vi "pickOffensiveTeam.vi"(0 "OffensiveTeam in":refnum<class "Ally.lvclass">, 1 "Game":refnum<class "Game.lvclass">, 5 "KeeperTeam":refnum<class "Ally.lvclass">, 7 "number_of_robots":i32, 9 "RobotRef":refnum<class "Robot.lvclass">[](array[class]), 11 "error in (no error)":errorcluster) -> (4 "OffensiveTeam out":refnum<class "Ally.lvclass">, 6 "RobotRef":refnum<class "Robot.lvclass">[](array[class]), 15 "error out":errorcluster)   [LabVIEW 2024, in "Ally.lvclass"]
uses:
  Ally.lvclass
  C:/Users/ROBOIME3/Documents/GitHub/SSL_AI/Team_class/Team.lvclass
  Robot_class/Robot.lvclass
  C:/Users/ROBOIME3/Documents/GitHub/SSL_AI/Object_class/Object.lvclass
  Game_class/Game.lvclass
  Utilities_class/Utilities.lvclass
  Team_class/Team.lvclass/Team.ctl
  Team_class/KeeperPlay.ctl
  Team_class/OffensivePlay.ctl
  Game_class/Game.lvclass/Game.ctl
  Parameters_class/Parameters.lvclass/Parameters.ctl
  Events_class/Events.lvclass/Events.ctl
  Object_class/Object.lvclass/Object.ctl
  Ball_class/Ball.lvclass/Ball.ctl
  Robot_class/Robot.lvclass/Robot.ctl
  Controls/AllyTeam.ctl
  Robot_class/roles.ctl
  Zone_class/zones.ctl
  Ally.lvclass/Ally.ctl
  Referee_class/Referee.lvclass/Referee.ctl
  Playbook_class/Playbook.lvclass/Playbook.ctl
  5RobotsSkill_class/5RobotsSkill.lvclass
  EliminateEnum.ctl
  Object_class/Read x.vi
  Object_class/Read y.vi
  Robot_class/Read id.vi
  Team_class/Read RobotRef.vi
  Robot_class/Write role.vi
  Robot_class/Read role.vi
  Robot_class/Write Zone.vi
  Read currentBallZone.vi
  Write currentBallZone.vi
  Game_class/Read Parameters.lvclass.vi
  Game_class/Read Referee.vi
  Referee_class/Read our_goalie_id.vi
  Parameters_class/Read minDistanceToPass.vi
  Playbook_class/Read offensive_plays.vi
  Object_class/Read position(x,y).vi
  Game_class/Read EnemyRef.vi
  Game_class/Read EventsRef.vi
  Game_class/Read BallRef.vi
  Game_class/Read OffensiveTeam.vi
  Game_class/Read NewParameters.vi
  Team_class/Read OffensivePlay.vi
  Ball_class/Read v_x.vi
  Ball_class/Read v_y.vi
  Events_class/Read ball_out_of_vision.vi
  Parameters_class/Read Number of Offesnive.vi
  Team_class/Write RobotRef.vi
  Team_class/Read KeeperPlay.vi
  Ball_class/Ball.lvclass
  Parameters_class/Parameters.lvclass
  Enemy_class/Enemy.lvclass
  Events_class/Events.lvclass
  Playbook_class/Playbook.lvclass
  Play_class/Play.lvclass
  TestPlay_class/TestPlay.lvclass
  EnemyPossessionAtEnemyFieldPlay_class/EnemyPossessionAtEnemyFieldPlay.lvclass
  EnemyPossessionAtOurFieldPlay_class/EnemyPossessionAtOurFieldPlay.lvclass
  NormalGamePlay_class/NormalGamePlay.lvclass
  IndirectEnemyPlay_class/IndirectEnemyPlay.lvclass
  PrepareKickoffAllyPlay_class/PrepareKickoffAllyPlay.lvclass
  PrepareKickoffEnemyPlay_class/PrepareKickoffEnemyPlay.lvclass
  KickPenaltyAllyPlay_class/KickPenaltyAllyPlay.lvclass
  PreparePenaltyAllyPlay_class/PreparePenaltyAllyPlay.lvclass
  DirectEnemyPlay_class/DirectEnemyPlay.lvclass
  PreparePenaltyEnemyPlay_class/PreparePenaltyEnemyPlay.lvclass
  BallOutOfFieldPlay_class/BallOutOfFieldPlay.lvclass
  StopOffensivePlay_class/StopOffensivePlay.lvclass
  PassPlay_class/PassPlay.lvclass
  DirectKickPlay_class/DirectKickPlay.lvclass
  HaltPlay_class/HaltPlay.lvclass
  PreparePassPlay_class/PreparePassPlay.lvclass
  PassToStriker_class/PassToStriker.lvclass
  PassTo2ndStriker_class/PassTo2ndStriker.lvclass
  SimplePass_class/SimplePass.lvclass
  PrepareRollToPassPlay_class/PrepareRollToPassPlay.lvclass
  PrepareDoublePassPlay_class/PrepareDoublePassPlay.lvclass
  TableWith2ndStrikerPlay_class/TableWith2ndStrikerPlay.lvclass
  TableWithStrikerPlay_class/TableWithStrikerPlay.lvclass
  PrepareTriplePassPlay_class/PrepareTriplePassPlay.lvclass
  ABCPassPlay_class/ABCPassPlay.lvclass
  PreparePassInGame1_class/PreparePassInGame1.lvclass
  ACBPassPlay_class/ACBPassPlay.lvclass
  PrepareKeeperPassPlay_class/PrepareKeeperPassPlay.lvclass
  KeeperPassToStrikerPlay_class/KeeperPassToStrikerPlay.lvclass
  5RobotsNormalGamePlay_class/5RobotsNormalGamePlay.lvclass
  5RobotsPassGamePlay_class/5RobotsPassGamePlay.lvclass
  5RobotsKeeperGame_class/5RobotsKeeperGame.lvclass
  5PreparePassGamePlay_class/5PreparePassGamePlay.lvclass
  Referee_class/Referee.lvclass
  Zone_class/Zone.lvclass
  MarkerSkill_class/MarkerSkill.lvclass
  22333355-05bd-4891-b21a-8224ee90334a.vi
  Field_class/Field.lvclass
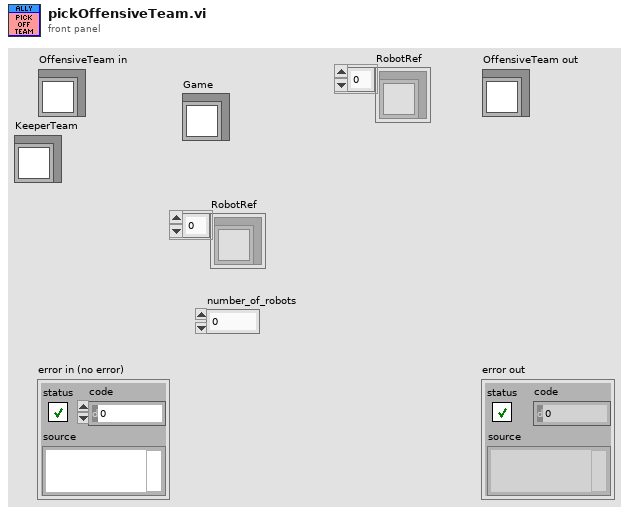
[diagram p1: front panel]
types:
  T1 = typedef "OffensivePlay.ctl" = enum16{"5RobotsPassGamePlay", "5PreparePassGame", "5RobotsKeeperGame", "KeeperPassToStriker", "5RobotsNormalGamePlay", "PrepareKeeperPass", "ACBPass", "ABCPass", "PrepareTriplePass", "TableWithStriker", "TableWith2ndStrikerPlay", "PrepareDoublePass", "PrepareRollToPass", "SimplePass", "PreparePass", "PassToStriker", "BallOutOfField", "PassTo2ndStriker", "StopOffensive", "Prepare Penalty Enemy", "EnemyPossessionAtEnemyField", "EnemyPossesionAtOurField", "TestPlay", "PreparePenaltyAlly", "KickPenaltyAlly", "PrepareKickoffAlly", "PrepareKickoffEnemy", "IndirectEnemy", "DirectEnemy", "PreparePassInGame1", "NormalGame", "DirectKick", "Pass", "Halt", "Timeout", "PassPlay", "PenaltyEnemy"}
  T2 = typedef "KeeperPlay.ctl" = enum16{"SimpleBallPlacementAlly", "BallPlacementAlly", "BallPlacementEnemy", "ZigZag", "Goto", "NormalGame", "KeeperPlay", "Halt", "Timeout", "PenaltyEnemy", "TestPlay"}
  T3 = enum16{"6", "5", "4", "3", "2", "1", "0", "Auto"}
  T4 = typedef "AllyTeam.ctl" = enum16{"Keeper", "Defender", "Attacker"}
  T5 = typedef "roles.ctl" = enum16{"SimpleBallPlacement", "BallPlacementAllyPasser", "BallPlacementAllyReceiver", "BallPlacementEnemy", "5Robots5th", "PassBestReceiver", "5Robots4th", "5Robots3rd", "5Robots2nd", "5Robots1st", "PassBestRobot", "WaitPass", "ABCThirdKicker", "ABCFirstKicker", "ABCSecondKicker", "Tabler", "TableFinalizer", "PrepareRollToPassRoller", "PrepareRollToPassReceiver", "SimplePassRoll", "SimplePassRollReceiver", "PenaltyDefense", "PreparePassReceiver 2", "PreparePassReceiver 1", "PassObserver", "Timeout", "Goto", "ZigZag", "None", "BallOutOfField", "DefenderArea", "Duelist", "AttackerStop", "FollowAttacker", "KeeperRole", "KickPenalty", "AttackerAimGoal", "AttackerBlock", "Marker", "Halt", "Shoot", "PassKicker", "PassReceiver", "TestRole", "PenaltyAttacker"}
  T6 = typedef "EliminateEnum.ctl" = enum16{"0", "1", "2"}
  T7 = typedef "Zone.lvclass/zones.ctl" = enum16{"Field", "LeftSide", "RightSide", "MidField", "LeftForward", "RightForward", "LeftMidField", "RightMidField", "LeftWing", "CenterForward", "RightWing", "Size"}
  T8 = typedef "NewParameters.ctl" = cluster{"PenaltyDistance":dbl, "DistanceAttackerToBackBall":dbl, "Division":enum16{"Div B", "Div A"}, "DistanceToAvoidyEnemyRobot":dbl, "BallPlacementDistance":dbl, "DisatanceBehindBallToStealBall":dbl, "MaxDistanceToPositionKickoff":dbl, "BlockEnemyTarget":bool, "MaxStopVAng":dbl, "DistanceMarkerToEnemy":dbl, "IgnoreDribblerContact":bool, "DistanceToBeginEnemyPosession":dbl, "GoToBallWhenEnemyNotMoving":bool, "EnemyDistanceToReduceVelocity":dbl, "TurnOnEnemyDistanceToReduceVelocity":bool, "EnemyDistanceToShootOutBall":dbl, "DefenseKickBall":bool, "MoreKickToGoal? (0-0.3)":dbl, "ChipKickInEnemyField":bool, "ShootOutRobotId":dbl, "FieldLenghtDenominatorInShootOut":dbl, "AdjustPositionInBallPlacement":bool, "PowerGodPass":dbl, "VelocityAbortEnemyPos":dbl, "MaxDistToBeginPass":dbl, "MinDistToBeginPass":dbl, "VelocityInDirects":dbl, "BadDribblerIDs":i32[], "NewKickToDistanceAroundBall":dbl, "PowerAvoidColisionMarker":dbl, "DistanceToAvoidColisionMarker":dbl, "AvoidBallKick":dbl, "DistanceTryKick":dbl, "SuicideKickDIstance":dbl, "AdjustFirstKickDistance":dbl, "AvoidAimLessKick":dbl, "DistanceToAvoidyEnemyShootRobot ":dbl, "NumberOfMarkers":dbl, "PotField":bool, "PIDLateral":bool, "MinDistanceFirstKickX":dbl, "MinDistanceFirstKickY":dbl, "FractionOfDistToTouchGround\nAfterChipKick":dbl, "FractionOfKickxWhen\nComposedWithKickz":dbl, "Style":T9, "MoveInTurnState":bool, "DistFromEnemyToConsider\nMoveInTurnState":dbl, "CascadePID":bool, "TurnAroundParameters":cluster{"Radius":dbl, "Multiplier":dbl, "ChordAngle":dbl}, "SafeDriveVel":dbl, "DistanceToGoToBackBall":dbl, "minDistanceToNotFinish\nEnemyPossession":dbl, "OneTouchShot":cluster{"angleFactor":dbl, "maxAngle":dbl, "Attack":bool, "Defense":bool}, "OpenAngleToGoal":cluster{"minAngle":dbl, "maxAngle":dbl, "minEvaluation":dbl}, "ShotInterception":cluster{"shotSpeed":dbl, "minEnemySpeed":dbl, "maxEnemySpeed":dbl, "minEvaluation":dbl}, "AllyTeamArray":T4[], "maxDefendersNumber":i32, "Zone":cluster{"GuardPositionArray":dbl[][], "ZoneMidField":dbl[], "CenterForwardWidth":dbl}, "MinEvaluationToShoot":dbl, "PassInterception":cluster{"maxPassSpeed":dbl, "minPassSpeed":dbl, "minEnemySpeed":dbl, "chipPassDistance":dbl, "chipPassEvaluation":dbl, "minEvaluation":dbl, "maxEnemySpeed":dbl}, "PassDistance":cluster{"maxDistance":dbl, "minDistance":dbl}, "receiverSpeed":dbl, "maxBallSpeed":dbl, "slackTime":dbl, "Turning radius":dbl, "Turning v_ang":dbl, "AlignError":cluster{"Distance":dbl, "Orientation":dbl, "V_norm(m/s)":dbl, "V_ang (rad/s)":dbl}, "RobotRadius":dbl, "KickerDistance":dbl, "keeper angle  to cover goalpost":dbl, "a_slide":dbl, "a_roll":dbl, "k_switch":dbl, "Penalty":u16}
  T9 = typedef "Style.ctl" = enum16{"Insanity", "Offensive", "Defensive"}
  T10 = typedef "offensive_plays.ctl" = cluster{"Play":refnum<class "Play.lvclass">, "TestPlay":refnum<class "TestPlay.lvclass">, "EnemyPossessionAtEnemyFieldPlay":refnum<class "EnemyPossessionAtEnemyFieldPlay.lvclass">, "EnemyPossessionAtOurFieldPlay":refnum<class "EnemyPossessionAtOurFieldPlay.lvclass">, "NormalGamePlay":refnum<class "NormalGamePlay.lvclass">, "IndirectEnemyPlay":refnum<class "IndirectEnemyPlay.lvclass">, "PrepareKickoffAllyPlay":refnum<class "PrepareKickoffAllyPlay.lvclass">, "PrepareKickoffEnemyPlay":refnum<class "PrepareKickoffEnemyPlay.lvclass">, "KickPenaltyAllyPlay":refnum<class "KickPenaltyAllyPlay.lvclass">, "PreparePenaltyAllyPlay":refnum<class "PreparePenaltyAllyPlay.lvclass">, "DirectEnemyPlay":refnum<class "DirectEnemyPlay.lvclass">, "PreparePenaltyEnemyPlay":refnum<class "PreparePenaltyEnemyPlay.lvclass">, "BallOutOfFieldPlay":refnum<class "BallOutOfFieldPlay.lvclass">, "StopOffensivePlay":refnum<class "StopOffensivePlay.lvclass">, "PassPlay":refnum<class "PassPlay.lvclass">, "DirectKickPlay":refnum<class "DirectKickPlay.lvclass">, "HaltPlay":refnum<class "HaltPlay.lvclass">, "PreparePassPlay":refnum<class "PreparePassPlay.lvclass">, "PassToStrikerPlay":refnum<class "PassToStriker.lvclass">, "PassTo2ndStrikerPlay":refnum<class "PassTo2ndStriker.lvclass">, "SimplePassPlay":refnum<class "SimplePass.lvclass">, "PrepareRollToPassPlay":refnum<class "PrepareRollToPassPlay.lvclass">, "PrepareDoublePassPlay":refnum<class "PrepareDoublePassPlay.lvclass">, "TableWith2ndStrikerPlay":refnum<class "TableWith2ndStrikerPlay.lvclass">, "TableWithStrikerPlay":refnum<class "TableWithStrikerPlay.lvclass">, "PrepareTriplePassPlay":refnum<class "PrepareTriplePassPlay.lvclass">, "ABCPassPlay":refnum<class "ABCPassPlay.lvclass">, "PreparePassInGame1":refnum<class "PreparePassInGame1.lvclass">, "ACBPassPlay":refnum<class "ACBPassPlay.lvclass">, "PrepareKeeperPassPlay":refnum<class "PrepareKeeperPassPlay.lvclass">, "KeeperPassToStrikerPlay":refnum<class "KeeperPassToStrikerPlay.lvclass">, "SimplePass":refnum<class "SimplePass.lvclass">, "SimplePass 2":refnum<class "SimplePass.lvclass">, "5RobotsNormalGamePlay":refnum<class "5RobotsNormalGamePlay.lvclass">, "5RobotsPassGamePlay":refnum<class "5RobotsPassGamePlay.lvclass">, "5RobotsKeeperGame":refnum<class "5RobotsKeeperGame.lvclass">, "5PreparePassGamePlay":refnum<class "5PreparePassGamePlay.lvclass">}
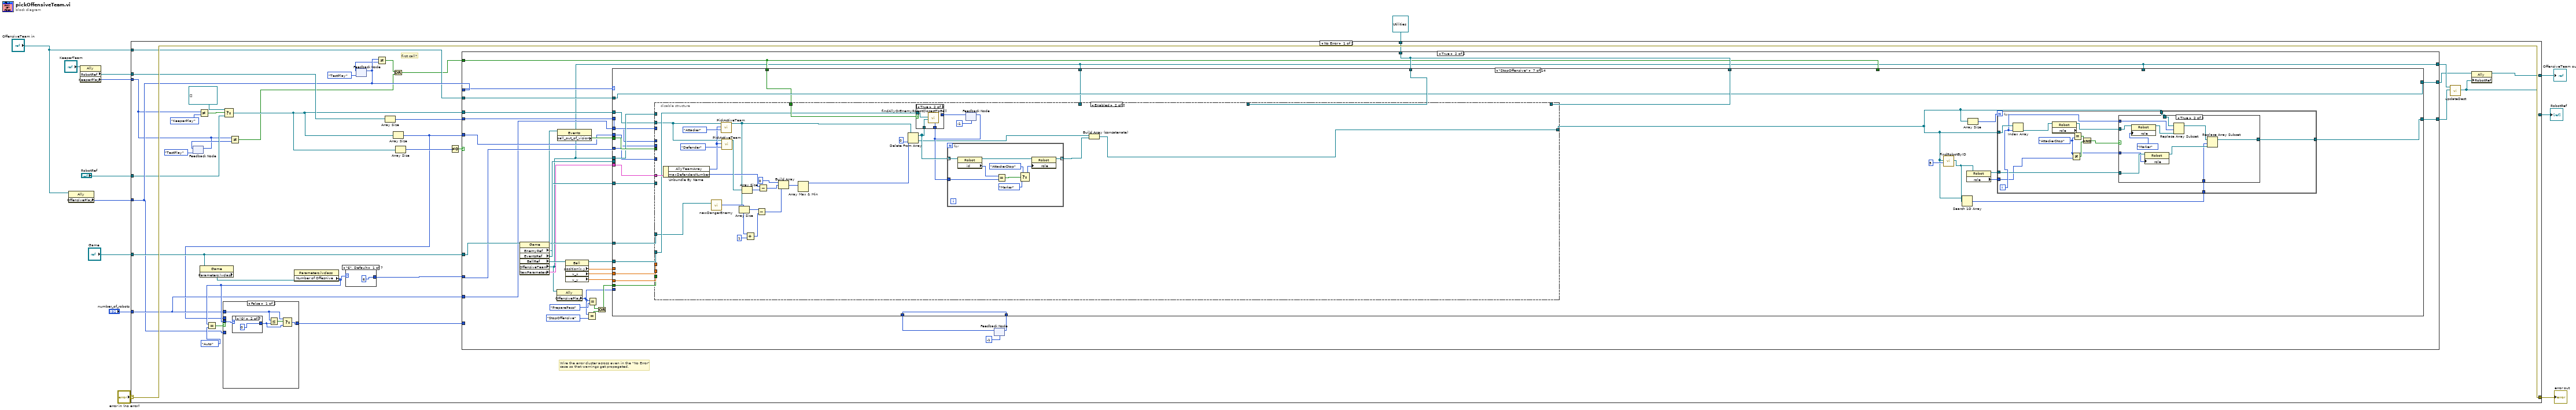
[diagram p0: block diagram]
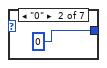
[diagram p2: hidden frame]
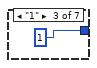
[diagram p3: hidden frame]
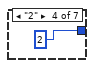
[diagram p4: hidden frame]
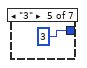
[diagram p5: hidden frame]
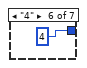
[diagram p6: hidden frame]
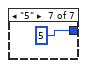
[diagram p7: hidden frame]
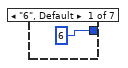
[diagram p8: hidden frame]
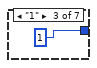
[diagram p9: hidden frame]
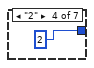
[diagram p10: hidden frame]
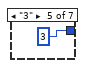
[diagram p11: hidden frame]
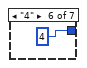
[diagram p12: hidden frame]
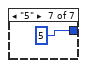
[diagram p13: hidden frame]
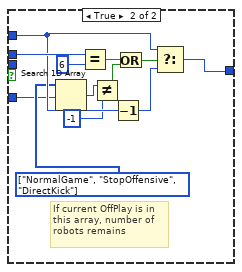
[diagram p14: hidden frame]
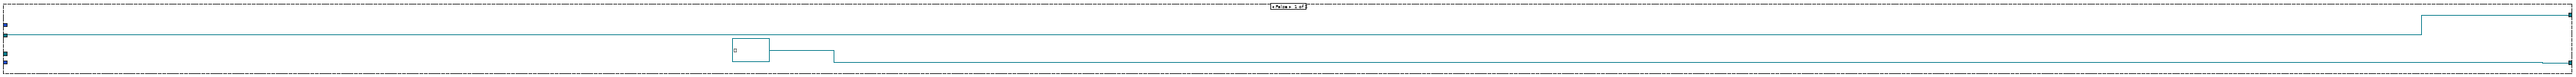
[diagram p15: hidden frame]
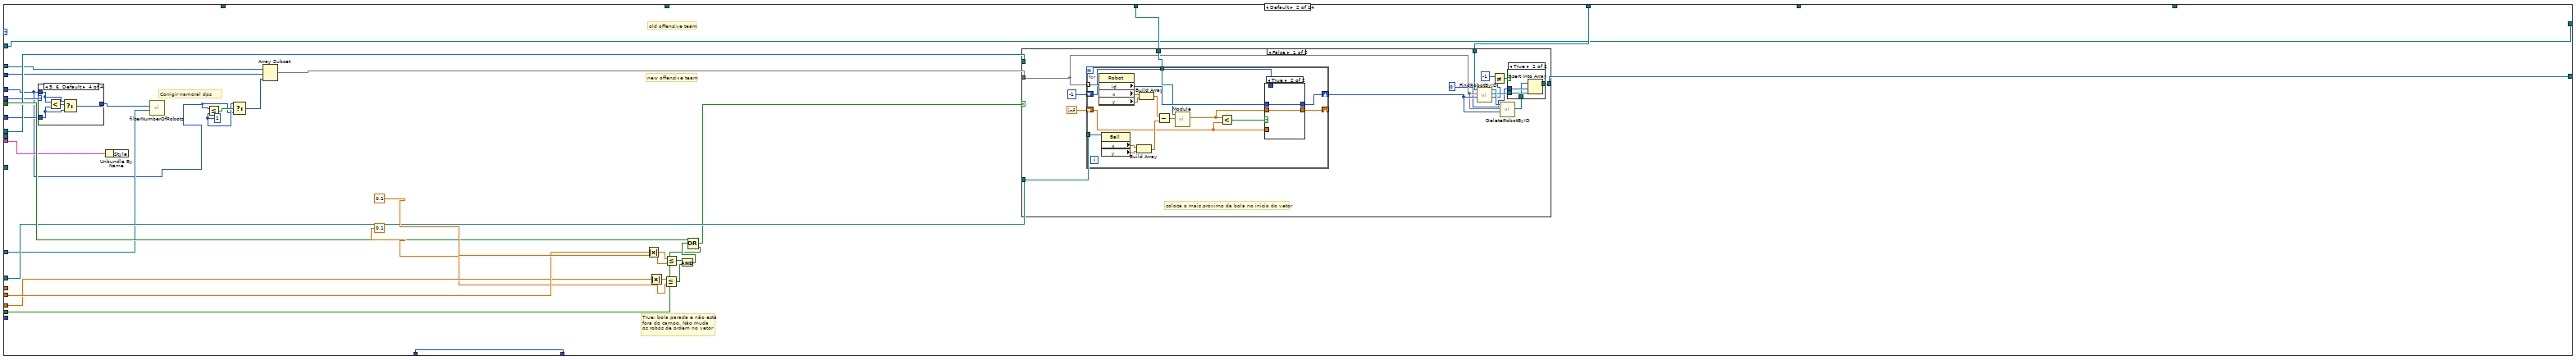
[diagram p17: hidden frame]
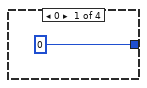
[diagram p18: hidden frame]
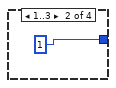
[diagram p19: hidden frame]
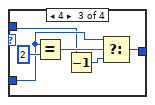
[diagram p20: hidden frame]
diagram:
  n1 = property class="Ally"(reference="OffensiveTeam in") -> ("OffensivePlay"=w2:T1)  [unwired: 1 in, 2 out]
  n2 = property class="Ally"(reference="KeeperTeam") -> ("RobotRef"=w7:refnum<class "Robot.lvclass">[], "KeeperPlay"=w1:T2)  [unwired: 1 in, 2 out]
  n3 = case shown="No Error" "error in (no error)" {
    selector: "error in (no error)" -> [w48 w2386]
    tunnel: [w48 w2386] -> w11
    tunnel: [w47 w2385] -> w13
    tunnel: "OffensiveTeam in" -> [w21 w2385]
    tunnel: "RobotRef" -> [w23 _]
    tunnel: "number_of_robots" -> [w30 _]
    tunnel: w7 -> [w46 _]
    tunnel: [w37 _] -> w6
    tunnel: "Game" -> [w41 _]
    tunnel: refnum<class "Utilities.lvclass"> refnum ("Utilities in") -> [w45 _]
    tunnel: w2 -> [w28 _]
    tunnel: w1 -> [w14 _]
    frame No Error {
      # "first call?"
      # "Wire the error cluster across even in the \"No Error\"\ncase so that warnings get propagated."
      n4 = feedback #1(OffensivePlay."TestPlay" ("OffensivePlay")) -> (w19:u16)
      n5 = feedback-in #1(w14) -> ()
      n6 = Not Equal?(x=w14, y=KeeperPlay."KeeperPlay") -> (x != y?=w24:bool)
      n7 = property class="Game"(reference=w41) -> ("Parameters.lvclass"=w40:refnum<class "Parameters.lvclass">)  [unwired: 1 in, 2 out]
      n8 = Select(t=refnum<class "Robot.lvclass">[] [] ("Array"), s=w24, f=w23) -> (s? t:f=w22:refnum<class "Robot.lvclass">[])
      n9 = Not Equal?(x=w14, y=w19) -> (x != y?=w17:bool)
      n10 = property class="Parameters.lvclass"(reference=w40) -> ("Number of Offesnive"=w32:T3)  [unwired: 1 in, 2 out]
      n11 = Equal?(x=w32, y=T3."Auto") -> (x = y?=w33:bool)
      n12 = case shown="\"6\", Default" w32 {
        tunnel: [6 0 1 2 3 4 5] -> w31
        frame "6", Default {
        }
        frame "0" {
        }
        frame "1" {
        }
        frame "2" {
        }
        frame "3" {
        }
        frame "4" {
        }
        frame "5" {
        }
      }
      n13 = feedback #2(OffensivePlay."TestPlay" ("OffensivePlay")) -> (w27:T1)
      n14 = feedback-in #2(w28) -> ()
      n15 = Not Equal?(x=w28, y=w27) -> (x != y?=w16:bool)
      n16 = Array Size(array=w46) -> (size(s)=w42:i32)
      n17 = Or(x=w16, y=w17) -> (x .or. y?=w15:bool)
      n18 = Array Size(array=w22) -> (size(s)=w29:i32)
      n19 = case shown="False" w33 {
        tunnel: w29 -> [_ w79]
        tunnel: w30 -> [w58 w77]
        tunnel: [w59 w75] -> w38
        tunnel: w32 -> [w60 _]
        tunnel: w28 -> [_ w68]
        frame False {
          n20 = case shown="\"0\"" w60 {
            tunnel: [6 0 1 2 3 4 5] -> w57
            frame "6", Default {
            }
            frame "0" {
            }
            frame "1" {
            }
            frame "2" {
            }
            frame "3" {
            }
            frame "4" {
            }
            frame "5" {
            }
          }
          n21 = Less Or Equal?(x=w58, y=w57) -> (x <= y?=w56:bool)
          n22 = Select(t=w58, s=w56, f=w57) -> (s? t:f=w59:i32)
        }
        frame True {
          w69 = T1[] [enum."NormalGame", enum."StopOffensive", enum."DirectKick"] items=["5RobotsPassGamePlay", "5PreparePassGame", "5RobotsKeeperGame", "KeeperPassToStriker", "5RobotsNormalGamePlay", "PrepareKeeperPass", "ACBPass", "ABCPass", "PrepareTriplePass", "TableWithStriker", "TableWith2ndStrikerPlay", "PrepareDoublePass", "PrepareRollToPass", "SimplePass", "PreparePass", "PassToStriker", "BallOutOfField", "PassTo2ndStriker", "StopOffensive", "Prepare Penalty Enemy", "EnemyPossessionAtEnemyField", "EnemyPossesionAtOurField", "TestPlay", "PreparePenaltyAlly", "KickPenaltyAlly", "PrepareKickoffAlly", "PrepareKickoffEnemy", "IndirectEnemy", "DirectEnemy", "PreparePassInGame1", "NormalGame", "DirectKick", "Pass", "Halt", "Timeout", "PassPlay", "PenaltyEnemy"] ("Array")
          # "If current OffPlay is in\nthis array, number of\nrobots remains"
          n23 = Search 1D Array(1D array=w69, element=w68) -> (index of element=w71:i32)  [unwired: 1 in]
          n24 = Equal?(x=w79, y=6) -> (x = y?=w74:bool)
          n25 = Not Equal?(x=w71, y=-1) -> (x != y?=w72:bool)
          n26 = Decrement(x=w77) -> (x-1=w76:i32)
          n27 = Or(x=w74, y=w72) -> (x .or. y?=w73:bool)
          n28 = Select(t=w77, s=w73, f=w76) -> (s? t:f=w75:i32)
        }
      }
      n29 = Array Size(array=w22) -> (size(s)=w43:i32)
      n30 = Not Equal To 0?(x=w43) -> (x != 0?=w44:bool)
      n31 = case shown="True" w44 {
        tunnel: w38 -> [_ _]
        tunnel: w22 -> [_ w98]
        tunnel: w42 -> [_ w97]
        tunnel: w28 -> [_ w113]
        tunnel: [refnum<class "Robot.lvclass">[] [] w112] -> w36
        tunnel: w41 -> [_ w111]
        tunnel: w45 -> [_ w105]
        tunnel: w15 -> [_ w91]
        tunnel: [_ w82] -> w35
        tunnel: w31 -> [_ w96]
        tunnel: w30 -> [_ w94]
        tunnel: w29 -> [_ w95]
        tunnel: w21 -> [w80 w88]
        tunnel: [w80 w86] -> w20
        frame False {
        }
        frame True {
          n32 = property class="Game"(reference=w111) -> (reference out=w92:refnum<class "Game.lvclass">, "EnemyRef"=w90:refnum<class "Enemy.lvclass">, "EventsRef"=w93:refnum<class "Events.lvclass">, "BallRef"=w110:refnum<class "Ball.lvclass">, "OffensiveTeam"=w82:refnum<class "Ally.lvclass">, "NewParameters"=w89:T8)  [unwired: 1 in, 1 out]
          n33 = property class="Ally"(reference=w82) -> ("OffensivePlay"=w101:T1)  [unwired: 1 in, 2 out]
          n34 = property class="Events"(reference=w93) -> ("ball_out_of_vision"=w107:bool)  [unwired: 1 in, 2 out]
          n35 = property class="Ball"(reference=w110) -> (reference out=w106:refnum<class "Ball.lvclass">, "position(x,y)"=w87:dbl[], "v_x"=w109:dbl, "v_y"=w108:dbl)  [unwired: 1 in, 1 out]
          n36 = Equal?(x=w101, y=OffensivePlay."StopOffensive") -> (x = y?=w99:bool)
          n37 = Equal?(x=w101, y=OffensivePlay."PreparePass") -> (x = y?=w103:bool)
          n38 = Or(x=w103, y=w99) -> (x .or. y?=w102:bool)
          n39 = feedback #3(-1) -> (w84:i32)
          n40 = case shown="\"StopOffensive\"" w113 {
            selector: w113 -> [_ _ _ _ _ _ _ w1611 _ _ w2011 _ _ _]
            tunnel: [w116 w134 w247 w522 w796 w1051 w1295 w1613 w1822 w1912 w2005 w2067 w2143 w2289] -> w112
            tunnel: w109 -> [_ w142 w252 w527 w801 w1056 w1320 _ _ _ _ _ w2162 w2315]
            tunnel: w108 -> [_ w141 w251 w526 w800 w1055 w1319 _ _ _ _ _ w2160 w2313]
            tunnel: w107 -> [_ w138 w250 w525 w799 w1054 w1318 _ _ _ _ _ _ _]
            tunnel: w106 -> [_ w137 w238 w513 w787 w1042 w1307 w1615 w1810 w1913 _ _ w2144 _]
            tunnel: w105 -> [_ w136 w249 w524 w798 w1053 w1317 w1614 _ _ _ _ w2158 w2297]
            tunnel: w105 -> [_ w135 w248 w523 w797 w1052 w1316 _ _ _ _ _ _ _]
            tunnel: w82 -> [_ w133 w246 w521 w795 w1050 w1315 w1607 w1818 w1908 _ _ w2129 _]
            tunnel: w102 -> [_ w132 w245 w520 w794 w1049 w1314 _ _ _ _ _ _ _]
            tunnel: w101 -> [_ _ _ _ _ _ _ _ _ _ _ _ _ _]
            tunnel: w91 -> [_ _ _ _ _ _ _ _ _ _ _ _ w2150 _]
            tunnel: w98 -> [w116 w130 w244 w519 w793 w1048 w1313 w1620 w1823 w1914 w2019 w2080 w2141 w2340]
            tunnel: w97 -> [_ w129 w243 w518 w792 w1047 w1312 w1619 _ _ _ _ _ w2339]
            tunnel: w96 -> [_ w127 w242 w517 w791 w1046 w1311 w1616 _ _ _ _ _ w2336]
            tunnel: w95 -> [_ w126 w241 w516 w790 w1045 w1310 w1617 _ _ _ _ _ w2337]
            tunnel: w94 -> [_ w119 w240 w515 w789 w1044 w1309 w1618 _ _ _ _ _ w2338]
            tunnel: w93 -> [_ _ _ _ _ _ _ _ _ _ _ _ _ _]
            tunnel: w92 -> [_ w121 w237 w512 w786 w1041 w1306 w1612 w1821 w1911 _ _ w2131 w2293]
            tunnel: w91 -> [_ _ w233 w508 _ _ w1302 w1610 _ _ _ _ _ _]
            tunnel: w90 -> [_ _ w239 w514 w788 w1043 w1308 _ _ _ _ _ _ _]
            tunnel: w89 -> [_ w123 w236 w511 w785 w1040 w1305 w1609 w1820 w1910 w2018 w2079 w2140 _]
            tunnel: w88 -> [w115 w118 w235 w510 w784 w1039 w1304 w1608 w1819 w1909 w2010 w2072 w2127 w2285]
            tunnel: w87 -> [_ _ _ _ _ _ _ w1606 w1817 w1907 _ _ _ _]
            tunnel: [w115 w118 w235 w510 w784 w1039 w1304 w1605 w1816 w1906 w2010 w2072 w2126 w2285] -> w86
            tunnel: w84 -> [w114 w117 w234 w509 w783 w1038 w1303 w1604 w1812 w1902 w2009 w2071 w2124 w2284]
            tunnel: [w114 w117 w234 w509 w783 w1038 w1303 w1604 w1813 w1902 w2009 w2071 w2124 w2284] -> w83
            tunnel: w82 -> [_ _ _ _ _ _ _ _ _ _ _ _ _ _]
            tunnel: w82 -> [_ _ _ _ _ _ w1301 _ _ _ _ _ _ _]
            frame "TestPlay" {
              # "Aqui entra a lógica para\nreeordenar o team de acordo \ncom quem deve assumir cada\nrole"
            }
            frame Default {
              w124 = 1 ("y")
              # "Corrigir namoral dps"
              # "old offensive team"
              # "new offensive team"
              # "True: bola parada e não está \nfora do campo. Não muda\nos robôs de ordem no vetor"
              n41 = case shown="5, 6, Default" w126 {
                tunnel: [0 ("number_of_robots") 1 w151 w158] -> w122
                tunnel: w127 -> [_ _ w153 w157]
                tunnel: w119 -> [_ _ w150 w156]
                frame 0 {
                }
                frame 1..3 {
                }
                frame 4 {
                  n42 = Equal?(x=w153, y=2) -> (x = y?=w154:bool)
                  n43 = Decrement(x=w150) -> (x-1=w152:i32)
                  n44 = Select(t=w153, s=w154, f=w152) -> (s? t:f=w151:i32)
                }
                frame 5, 6, Default {
                  n45 = Less?(x=w156, y=w157) -> (x < y?=w159:bool)
                  n46 = Select(t=w156, s=w159, f=w157) -> (s? t:f=w158:i32)
                }
              }
              n47 = Unbundle By Name(w123) -> ()  [unwired: 1 out]
              n48 = call "filterNumberOfRobots.vi"("Game"=w121, "previousNumberOfRobots"=w122) -> ()  [unwired: 7 in, 3 out]
              n49 = Less Or Equal?(x=w119, y=w124) -> (x <= y?=w125:bool)
              n50 = Select(t=w124, s=w125, f=w119) -> (s? t:f=w120:i32)
              n51 = Array Subset(array=w130, index=w129, length=w120) -> (w128:refnum<class "Robot.lvclass">[])
              n52 = Absolute Value(x=w142) -> (abs(x)=w146:dbl)
              n53 = Absolute Value(x=w141) -> (abs(x)=w145:dbl)
              n54 = Less Or Equal?(x=w145, y=0.1) -> (x <= y?=w143:bool)
              n55 = Less Or Equal?(x=w146, y=0.1) -> (x <= y?=w144:bool)
              n56 = Compound Arithmetic op=AND(w144, w143) -> (w139:bool)
              n57 = Compound Arithmetic op=OR(w138, w139, w132) -> (w131:bool)
              n58 = case shown="False" w131 {
                tunnel: w137 -> [w174 _]
                tunnel: w136 -> [w172 w204]
                tunnel: w135 -> [w171 _]
                tunnel: w128 -> [w167 w207]
                tunnel: [w165 w201] -> w134
                tunnel: w133 -> [_ w206]
                frame False {
                  # "coloca o mais próximo da bola no inicio do vetor"
                  n59 = for {
                    tunnel: w167 -> [w196] mode=indexing
                    tunnel: w174 -> [w195]
                    shift-right: [w186] -> w170
                    shift-left: -1 ("id") -> [w182]
                    shift-right: [w184] -> _
                    shift-left: inf -> [w181]
                    tunnel: w172 -> [w180]
                    n60 = property class="Robot"(reference=w196) -> ("id"=w185:i32, "x"=w194:dbl, "y"=w193:dbl)  [unwired: 1 in, 2 out]
                    n61 = property class="Ball"(reference=w195) -> ("x"=w192:dbl, "y"=w191:dbl)  [unwired: 1 in, 2 out]
                    n62 = Build Array(w192, w191) -> (w189:dbl[])
                    n63 = Build Array(w194, w193) -> (w190:dbl[])
                    n64 = Subtract(x=w190, y=w189) -> (x-y=w188:dbl[])
                    n65 = call "Module.vi"("2D vector"=w188, "Utilities in"=w180) -> ("Modulo"=w183:dbl)  [unwired: 7 in, 2 out]
                    n66 = Less?(x=w183, y=w181) -> (x < y?=w187:bool)
                    n67 = case shown="True" w187 {
                      tunnel: [w198 w200] -> w186
                      tunnel: w185 -> [_ w200]
                      tunnel: [w197 w199] -> w184
                      tunnel: w183 -> [_ w199]
                      tunnel: w182 -> [w198 _]
                      tunnel: w181 -> [w197 _]
                      frame False {
                      }
                      frame True {
                      }
                    }
                  }
                  n68 = call "FindRobotByID.vi"("id"=w170, "RobotRef"=w167, "Utilities in"=w171) -> ("index"=w162:i32, "Robot"=w168:refnum<class "Robot.lvclass">, "Utilities out"=w169:refnum<class "Utilities.lvclass">)  [unwired: 5 in, 1 out]
                  n69 = Not Equal?(x=-1, y=w162) -> (x != y?=w160:bool)
                  n70 = call "DeleteRobotByID.vi"("id"=w170, "RobotRef"=w167, "Utilities in"=w169) -> ("RobotRef out"=w164:refnum<class "Robot.lvclass">[])  [unwired: 6 in, 2 out]
                  n71 = case shown="True" w160 {
                    tunnel: w168 -> [_ w179]
                    tunnel: 0 ("index") -> [_ w178]
                    tunnel: [w175 w177] -> w165
                    tunnel: w164 -> [w175 w176]
                    frame False {
                    }
                    frame True {
                      n72 = Insert Into Array(array=w176, index=w178, new element=w179) -> (w177:refnum<class "Robot.lvclass">[])
                    }
                  }
                }
                frame True {
                  n73 = property class="Ally"(reference=w206) -> ("RobotRef"=w205:refnum<class "Robot.lvclass">[])  [unwired: 1 in, 2 out]
                  n74 = for {
                    shift-right: [w209] -> w202
                    shift-left: w207 -> [w212]
                    shift-right: [w210] -> w203
                    shift-left: refnum<class "Robot.lvclass">[] [] -> [w213]
                    tunnel: w205 -> [w214] mode=indexing
                    tunnel: w204 -> [w211]
                    n75 = property class="Robot"(reference=w214) -> ("id"=w219:i32)  [unwired: 1 in, 2 out]
                    n76 = call "FindRobotByID.vi"("id"=w219, "RobotRef"=w212, "Utilities in"=w211) -> ("index"=w216:i32, "Robot"=w220:refnum<class "Robot.lvclass">, "Utilities out"=w218:refnum<class "Utilities.lvclass">)  [unwired: 5 in, 1 out]
                    n77 = Equal?(x=w216, y=-1) -> (x = y?=w217:bool)
                    n78 = case shown="False" w217 {
                      tunnel: w220 -> [w221 _]
                      tunnel: [w227 w229] -> w210
                      tunnel: w213 -> [w226 w229]
                      tunnel: w212 -> [w225 w228]
                      tunnel: w219 -> [w224 _]
                      tunnel: [w223 w228] -> w209
                      tunnel: w218 -> [w222 _]
                      tunnel: w214 -> [_ _]
                      frame False {
                        n79 = Insert Into Array(array=w226, new element=w221) -> (w227:refnum<class "Robot.lvclass">[])  [unwired: 1 in]
                        n80 = call "DeleteRobotByID.vi"("id"=w224, "RobotRef"=w225, "Utilities in"=w222) -> ("RobotRef out"=w223:refnum<class "Robot.lvclass">[])  [unwired: 6 in, 2 out]
                      }
                      frame True {
                      }
                    }
                  }
                  n81 = for {
                    shift-right: [w230] -> w201
                    shift-left: w203 -> [w232]
                    tunnel: w202 -> [w231] mode=indexing
                    n82 = Insert Into Array(array=w232, new element=w231) -> (w230:refnum<class "Robot.lvclass">[])  [unwired: 1 in]
                  }
                }
              }
            }
            frame "EnemyPossesionAtOurField" {
              # "old offensive team"
              n83 = disable-structure shown="Enabled" {
                disable-tunnel: w252 -> [w286 _]
                disable-tunnel: w251 -> [w285 _]
                disable-tunnel: w250 -> [w282 _]
                disable-tunnel: w249 -> [w281 _]
                disable-tunnel: w248 -> [w280 _]
                disable-tunnel: [w279 w485] -> w247
                disable-tunnel: w246 -> [w278 _]
                disable-tunnel: w245 -> [w277 _]
                disable-tunnel: w244 -> [w276 w493]
                disable-tunnel: w243 -> [w275 _]
                disable-tunnel: w242 -> [w273 _]
                disable-tunnel: w241 -> [w272 _]
                disable-tunnel: w240 -> [w271 _]
                disable-tunnel: w239 -> [w270 _]
                disable-tunnel: w238 -> [w268 w468]
                disable-tunnel: w237 -> [w260 w475]
                disable-tunnel: w236 -> [w259 w494]
                disable-tunnel: w233 -> [_ w470]
                frame Disabled {
                  w255 = 1 ("y")
                  # "Deve trocar quem vai pra bola\nquando trocar robô inimigo mais\nperto da bola"
                  # "new offensive team"
                  # "True: bola parada e não está \nfora do campo. Não muda\nos robôs de ordem no vetor"
                  n84 = case shown="0" w272 {
                    tunnel: [0 ("number_of_robots") 1 w295 w302] -> w261
                    tunnel: w273 -> [_ _ w297 w301]
                    tunnel: w271 -> [_ _ w294 w300]
                    frame 0 {
                    }
                    frame 1..3 {
                    }
                    frame 4 {
                      n85 = Equal?(x=w297, y=2) -> (x = y?=w298:bool)
                      n86 = Decrement(x=w294) -> (x-1=w296:i32)
                      n87 = Select(t=w297, s=w298, f=w296) -> (s? t:f=w295:i32)
                    }
                    frame 5, 6, Default {
                      n88 = Less?(x=w300, y=w301) -> (x < y?=w303:bool)
                      n89 = Select(t=w300, s=w303, f=w301) -> (s? t:f=w302:i32)
                    }
                  }
                  n90 = Unbundle By Name(w259) -> ("Style"=w257:T9)
                  n91 = property class="Enemy"(reference=w270) -> ("RobotRef"=w269:refnum<class "Robot.lvclass">[])  [unwired: 1 in, 2 out]
                  n92 = call "filterNumberOfRobots.vi"("Game"=w260, "previousNumberOfRobots"=w261) -> ("finalNumberOfRobots"=w258:i32)  [unwired: 7 in, 2 out]
                  n93 = call "findAllyOrEnemyRobotClosestToBall.vi"("Ally/Enemy Robots"=w269, "Ball"=w268) -> ("Robot"=w267:refnum<class "Robot.lvclass">)  [unwired: 5 in, 4 out]
                  n94 = Subtract(x=w258, y=w257) -> (x-y=w254:i32)
                  n95 = Less Or Equal?(x=w254, y=w255) -> (x <= y?=w256:bool)
                  n96 = Select(t=w255, s=w256, f=w254) -> (s? t:f=w253:i32)
                  n97 = Array Subset(array=w276, index=w275, length=w253) -> (w274:refnum<class "Robot.lvclass">[])
                  n98 = property class="Robot"(reference=w267) -> (reference out=w262:refnum<class "Robot.lvclass">, "id"=w264:i32)  [unwired: 1 in, 1 out]
                  n99 = feedback #4(-1) -> (w266:i32)
                  n100 = Not Equal?(x=w264, y=w266) -> (x != y?=w263:bool)
                  n101 = feedback-in #4(w264) -> ()
                  n102 = Absolute Value(x=w286) -> (abs(x)=w290:dbl)
                  n103 = Absolute Value(x=w285) -> (abs(x)=w289:dbl)
                  n104 = Less Or Equal?(x=w289, y=0.1) -> (x <= y?=w287:bool)
                  n105 = Less Or Equal?(x=w290, y=0.1) -> (x <= y?=w288:bool)
                  n106 = Compound Arithmetic op=AND(w288, w287) -> (w283:bool)
                  n107 = Compound Arithmetic op=OR(w282, w283, w277) -> ()  [unwired: 1 out]
                  n108 = disable-structure shown="Enabled" {
                    disable-tunnel: w281 -> [w311 w389]
                    disable-tunnel: w280 -> [w310 w388]
                    disable-tunnel: [w309 w387] -> w279
                    disable-tunnel: w278 -> [w308 w393]
                    disable-tunnel: w274 -> [w307 w392]
                    disable-tunnel: w268 -> [w306 w390]
                    disable-tunnel: w263 -> [w305 _]
                    disable-tunnel: w262 -> [w304 w391]
                    disable-tunnel: w260 -> [_ w386]
                    frame Disabled {
                      n109 = case shown="True" w305 {
                        tunnel: w306 -> [_ _]
                        tunnel: w311 -> [w315 w357]
                        tunnel: w310 -> [_ w356]
                        tunnel: w307 -> [w318 w352]
                        tunnel: [w312 w350] -> w309
                        tunnel: w308 -> [w317 _]
                        tunnel: w304 -> [_ w344]
                        frame False {
                          n110 = property class="Ally"(reference=w317) -> ("RobotRef"=w316:refnum<class "Robot.lvclass">[])  [unwired: 1 in, 2 out]
                          n111 = for {
                            shift-right: [w320] -> w313
                            shift-left: w318 -> [w323]
                            shift-right: [w321] -> w314
                            shift-left: refnum<class "Robot.lvclass">[] [] -> [w324]
                            tunnel: w316 -> [w325] mode=indexing
                            tunnel: w315 -> [w322]
                            n112 = property class="Robot"(reference=w325) -> ("id"=w330:i32)  [unwired: 1 in, 2 out]
                            n113 = call "FindRobotByID.vi"("id"=w330, "RobotRef"=w323, "Utilities in"=w322) -> ("index"=w327:i32, "Robot"=w331:refnum<class "Robot.lvclass">, "Utilities out"=w329:refnum<class "Utilities.lvclass">)  [unwired: 5 in, 1 out]
                            n114 = Equal?(x=w327, y=-1) -> (x = y?=w328:bool)
                            n115 = case shown="False" w328 {
                              tunnel: w331 -> [w332 _]
                              tunnel: [w338 w340] -> w321
                              tunnel: w324 -> [w337 w340]
                              tunnel: w323 -> [w336 w339]
                              tunnel: w330 -> [w335 _]
                              tunnel: [w334 w339] -> w320
                              tunnel: w329 -> [w333 _]
                              tunnel: w325 -> [_ _]
                              frame False {
                                n116 = Insert Into Array(array=w337, new element=w332) -> (w338:refnum<class "Robot.lvclass">[])  [unwired: 1 in]
                                n117 = call "DeleteRobotByID.vi"("id"=w335, "RobotRef"=w336, "Utilities in"=w333) -> ("RobotRef out"=w334:refnum<class "Robot.lvclass">[])  [unwired: 6 in, 2 out]
                              }
                              frame True {
                              }
                            }
                          }
                          n118 = for {
                            shift-right: [w341] -> w312
                            shift-left: w314 -> [w343]
                            tunnel: w313 -> [w342] mode=indexing
                            n119 = Insert Into Array(array=w343, new element=w342) -> (w341:refnum<class "Robot.lvclass">[])  [unwired: 1 in]
                          }
                        }
                        frame True {
                          # "\"troca pesonalidade\""
                          # "coloca o nosso robô mais próximo do inimigo mais perto da bola no inicio do vetor"
                          n120 = for {
                            tunnel: w352 -> [w380] mode=indexing
                            tunnel: w344 -> [w379]
                            shift-right: [w370] -> w355
                            shift-left: -1 ("id") -> [w366]
                            shift-right: [w368] -> _
                            shift-left: inf -> [w365]
                            tunnel: w357 -> [w364]
                            n121 = property class="Robot"(reference=w379) -> ("x"=w376:dbl, "y"=w375:dbl)  [unwired: 1 in, 2 out]
                            n122 = property class="Robot"(reference=w380) -> ("id"=w369:i32, "x"=w378:dbl, "y"=w377:dbl)  [unwired: 1 in, 2 out]
                            n123 = Build Array(w376, w375) -> (w373:dbl[])
                            n124 = Build Array(w378, w377) -> (w374:dbl[])
                            n125 = Subtract(x=w374, y=w373) -> (x-y=w372:dbl[])
                            n126 = call "Module.vi"("2D vector"=w372, "Utilities in"=w364) -> ("Modulo"=w367:dbl)  [unwired: 7 in, 2 out]
                            n127 = Less?(x=w367, y=w365) -> (x < y?=w371:bool)
                            n128 = case shown="True" w371 {
                              tunnel: [w382 w384] -> w370
                              tunnel: w369 -> [_ w384]
                              tunnel: [w381 w383] -> w368
                              tunnel: w367 -> [_ w383]
                              tunnel: w366 -> [w382 _]
                              tunnel: w365 -> [w381 _]
                              frame False {
                              }
                              frame True {
                              }
                            }
                          }
                          n129 = call "FindRobotByID.vi"("id"=w355, "RobotRef"=w352, "Utilities in"=w356) -> ("index"=w347:i32, "Robot"=w353:refnum<class "Robot.lvclass">, "Utilities out"=w354:refnum<class "Utilities.lvclass">)  [unwired: 5 in, 1 out]
                          n130 = Not Equal?(x=-1, y=w347) -> (x != y?=w345:bool)
                          n131 = call "DeleteRobotByID.vi"("id"=w355, "RobotRef"=w352, "Utilities in"=w354) -> ("RobotRef out"=w349:refnum<class "Robot.lvclass">[])  [unwired: 6 in, 2 out]
                          n132 = case shown="False" w345 {
                            tunnel: w353 -> [_ w363]
                            tunnel: 0 ("index") -> [_ w362]
                            tunnel: [w359 w361] -> w350
                            tunnel: w349 -> [w359 w360]
                            frame False {
                            }
                            frame True {
                              n133 = Insert Into Array(array=w360, index=w362, new element=w363) -> (w361:refnum<class "Robot.lvclass">[])
                            }
                          }
                        }
                      }
                    }
                    frame Enabled {
                      n134 = case shown="True" TRUE {
                        tunnel: w390 -> [_ _]
                        tunnel: w389 -> [w397 w440]
                        tunnel: w388 -> [_ w439]
                        tunnel: w392 -> [w400 w435]
                        tunnel: [w394 w433] -> w387
                        tunnel: w393 -> [w399 _]
                        tunnel: w391 -> [_ _]
                        tunnel: w386 -> [_ w427]
                        frame False {
                          n135 = property class="Ally"(reference=w399) -> ("RobotRef"=w398:refnum<class "Robot.lvclass">[])  [unwired: 1 in, 2 out]
                          n136 = for {
                            shift-right: [w402] -> w395
                            shift-left: w400 -> [w405]
                            shift-right: [w403] -> w396
                            shift-left: refnum<class "Robot.lvclass">[] [] -> [w406]
                            tunnel: w398 -> [w407] mode=indexing
                            tunnel: w397 -> [w404]
                            n137 = property class="Robot"(reference=w407) -> ("id"=w412:i32)  [unwired: 1 in, 2 out]
                            n138 = call "FindRobotByID.vi"("id"=w412, "RobotRef"=w405, "Utilities in"=w404) -> ("index"=w409:i32, "Robot"=w413:refnum<class "Robot.lvclass">, "Utilities out"=w411:refnum<class "Utilities.lvclass">)  [unwired: 5 in, 1 out]
                            n139 = Equal?(x=w409, y=-1) -> (x = y?=w410:bool)
                            n140 = case shown="False" w410 {
                              tunnel: w413 -> [w414 _]
                              tunnel: [w420 w422] -> w403
                              tunnel: w406 -> [w419 w422]
                              tunnel: w405 -> [w418 w421]
                              tunnel: w412 -> [w417 _]
                              tunnel: [w416 w421] -> w402
                              tunnel: w411 -> [w415 _]
                              tunnel: w407 -> [_ _]
                              frame False {
                                n141 = Insert Into Array(array=w419, new element=w414) -> (w420:refnum<class "Robot.lvclass">[])  [unwired: 1 in]
                                n142 = call "DeleteRobotByID.vi"("id"=w417, "RobotRef"=w418, "Utilities in"=w415) -> ("RobotRef out"=w416:refnum<class "Robot.lvclass">[])  [unwired: 6 in, 2 out]
                              }
                              frame True {
                              }
                            }
                          }
                          n143 = for {
                            shift-right: [w423] -> w394
                            shift-left: w396 -> [w425]
                            tunnel: w395 -> [w424] mode=indexing
                            n144 = Insert Into Array(array=w425, new element=w424) -> (w423:refnum<class "Robot.lvclass">[])  [unwired: 1 in]
                          }
                        }
                        frame True {
                          # "Em vez do robo mais perto do inimigo mais perto da bola, pegamos simplesmente o mais proximo da bola"
                          # "\"troca pesonalidade\""
                          n145 = property class="Game"(reference=w427) -> ("BallRef"=w426:refnum<class "Ball.lvclass">)  [unwired: 1 in, 2 out]
                          n146 = for {
                            tunnel: w435 -> [w463] mode=indexing
                            tunnel: w426 -> [w462]
                            shift-right: [w453] -> w438
                            shift-left: -1 ("id") -> [w449]
                            shift-right: [w451] -> _
                            shift-left: inf -> [w448]
                            tunnel: w440 -> [w447]
                            n147 = property class="Robot"(reference=w463) -> ("id"=w452:i32, "x"=w461:dbl, "y"=w460:dbl)  [unwired: 1 in, 2 out]
                            n148 = property class="Ball"(reference=w462) -> ("x"=w459:dbl, "y"=w458:dbl)  [unwired: 1 in, 2 out]
                            n149 = Build Array(w459, w458) -> (w456:dbl[])
                            n150 = Build Array(w461, w460) -> (w457:dbl[])
                            n151 = Subtract(x=w457, y=w456) -> (x-y=w455:dbl[])
                            n152 = call "Module.vi"("2D vector"=w455, "Utilities in"=w447) -> ("Modulo"=w450:dbl)  [unwired: 7 in, 2 out]
                            n153 = Less?(x=w450, y=w448) -> (x < y?=w454:bool)
                            n154 = case shown="True" w454 {
                              tunnel: [w465 w467] -> w453
                              tunnel: w452 -> [_ w467]
                              tunnel: [w464 w466] -> w451
                              tunnel: w450 -> [_ w466]
                              tunnel: w449 -> [w465 _]
                              tunnel: w448 -> [w464 _]
                              frame False {
                              }
                              frame True {
                              }
                            }
                          }
                          n155 = call "FindRobotByID.vi"("id"=w438, "RobotRef"=w435, "Utilities in"=w439) -> ("index"=w430:i32, "Robot"=w436:refnum<class "Robot.lvclass">, "Utilities out"=w437:refnum<class "Utilities.lvclass">)  [unwired: 5 in, 1 out]
                          n156 = Not Equal?(x=-1, y=w430) -> (x != y?=w428:bool)
                          n157 = call "DeleteRobotByID.vi"("id"=w438, "RobotRef"=w435, "Utilities in"=w437) -> ("RobotRef out"=w432:refnum<class "Robot.lvclass">[])  [unwired: 6 in, 2 out]
                          n158 = case shown="False" w428 {
                            tunnel: w436 -> [_ w446]
                            tunnel: 0 ("index") -> [_ w445]
                            tunnel: [w442 w444] -> w433
                            tunnel: w432 -> [w442 w443]
                            frame False {
                            }
                            frame True {
                              n159 = Insert Into Array(array=w443, index=w445, new element=w446) -> (w444:refnum<class "Robot.lvclass">[])
                            }
                          }
                        }
                      }
                    }
                  }
                }
                frame Enabled {
                  n160 = Unbundle By Name(w494) -> ("AllyTeamArray"=w490:T4[], "maxDefendersNumber"=w487:i32)
                  n161 = call "newDangerEnemy.vi"("Game"=w475) -> ("numberOfPossible\nEnemiesToMark"=w476:i32)  [unwired: 11 in, 3 out]
                  n162 = call "PickActiveTeam.vi"("Robots"=w493, "AllyTeamArray"=w490, "Team"=AllyTeam."Attacker") -> ("Robots out"=w484:refnum<class "Robot.lvclass">[])  [unwired: 15 in, 1 out]
                  n163 = call "PickActiveTeam.vi"("Robots"=w493, "AllyTeamArray"=w490, "Team"=AllyTeam."Defender") -> ("Robots out"=w489:refnum<class "Robot.lvclass">[])  [unwired: 15 in, 1 out]
                  n164 = Array Size(array=w489) -> (size(s)=w486:i32)
                  n165 = Add(x=w476, y=1) -> (x+y=w474:i32)
                  n166 = Array Size(array=w484) -> (size(s)=w483:i32)
                  n167 = Subtract(x=w487, y=w486) -> (x-y=w481:i32)
                  n168 = Subtract(x=w483, y=w474) -> (x-y=w480:i32)
                  n169 = Build Array(0 ("y"), w481, w480) -> (w479:i32[])
                  n170 = Array Max & Min(array=w479) -> (max value=w478:i32)  [unwired: 3 out]
                  n171 = Delete From Array(array=w484, length=w478, index=0) -> (array with subset deleted=w471:refnum<class "Robot.lvclass">[])  [unwired: 1 out]
                  n172 = feedback #5(-1 ("y")) -> (w472:i32)
                  n173 = case shown="True" w470 {
                    tunnel: w471 -> [_ w498]
                    tunnel: w468 -> [_ w497]
                    tunnel: [w495 w496] -> w469
                    tunnel: w472 -> [w495 _]
                    frame False {
                    }
                    frame True {
                      n174 = call "findAllyOrEnemyRobotClosestToBall.vi"("Ally/Enemy Robots"=w498, "Ball"=w497) -> ("id"=w496:i32)  [unwired: 5 in, 4 out]
                    }
                  }
                  n175 = for {
                    tunnel: w471 -> [w507] mode=indexing
                    tunnel: w469 -> [w505]
                    tunnel: [w499] -> w485 mode=indexing
                    n176 = property class="Robot"(reference=w507) -> (reference out=w501:refnum<class "Robot.lvclass">, "id"=w506:i32)  [unwired: 1 in, 1 out]
                    n177 = Equal?(x=w506, y=w505) -> (x = y?=w504:bool)
                    n178 = Select(t=roles."Duelist" ("role"), s=w504, f=roles."Marker" ("role")) -> (s? t:f=w500:T5)
                    n179 = property class="Robot"(reference=w501, "role"=w500) -> (reference out=w499:refnum<class "Robot.lvclass">)  [unwired: 1 in, 1 out]
                  }
                  n180 = feedback-in #5(w469) -> ()
                }
              }
            }
            frame "DirectEnemy" {
              n181 = disable-structure shown="Enabled" {
                disable-tunnel: w527 -> [w561 _]
                disable-tunnel: w526 -> [w560 _]
                disable-tunnel: w525 -> [w557 _]
                disable-tunnel: w524 -> [w556 _]
                disable-tunnel: w523 -> [w555 _]
                disable-tunnel: [w554 w760] -> w522
                disable-tunnel: w521 -> [w553 _]
                disable-tunnel: w520 -> [w552 _]
                disable-tunnel: w519 -> [w551 w768]
                disable-tunnel: w518 -> [w550 _]
                disable-tunnel: w517 -> [w548 _]
                disable-tunnel: w516 -> [w547 _]
                disable-tunnel: w515 -> [w546 _]
                disable-tunnel: w514 -> [w545 _]
                disable-tunnel: w513 -> [w543 w746]
                disable-tunnel: w512 -> [w535 w750]
                disable-tunnel: w511 -> [w534 w769]
                disable-tunnel: w508 -> [_ w744]
                frame Disabled {
                  w530 = 1 ("y")
                  # "Deve trocar quem vai pra bola\nquando trocar robô inimigo mais\nperto da bola"
                  # "new offensive team"
                  # "True: bola parada e não está \nfora do campo. Não muda\nos robôs de ordem no vetor"
                  n182 = case shown="0" w547 {
                    tunnel: [0 ("number_of_robots") 1 w570 w577] -> w536
                    tunnel: w548 -> [_ _ w572 w576]
                    tunnel: w546 -> [_ _ w569 w575]
                    frame 0 {
                    }
                    frame 1..3 {
                    }
                    frame 4 {
                      n183 = Equal?(x=w572, y=2) -> (x = y?=w573:bool)
                      n184 = Decrement(x=w569) -> (x-1=w571:i32)
                      n185 = Select(t=w572, s=w573, f=w571) -> (s? t:f=w570:i32)
                    }
                    frame 5, 6, Default {
                      n186 = Less?(x=w575, y=w576) -> (x < y?=w578:bool)
                      n187 = Select(t=w575, s=w578, f=w576) -> (s? t:f=w577:i32)
                    }
                  }
                  n188 = Unbundle By Name(w534) -> ("Style"=w532:T9)
                  n189 = property class="Enemy"(reference=w545) -> ("RobotRef"=w544:refnum<class "Robot.lvclass">[])  [unwired: 1 in, 2 out]
                  n190 = call "filterNumberOfRobots.vi"("Game"=w535, "previousNumberOfRobots"=w536) -> ("finalNumberOfRobots"=w533:i32)  [unwired: 7 in, 2 out]
                  n191 = call "findAllyOrEnemyRobotClosestToBall.vi"("Ally/Enemy Robots"=w544, "Ball"=w543) -> ("Robot"=w542:refnum<class "Robot.lvclass">)  [unwired: 5 in, 4 out]
                  n192 = Subtract(x=w533, y=w532) -> (x-y=w529:i32)
                  n193 = Less Or Equal?(x=w529, y=w530) -> (x <= y?=w531:bool)
                  n194 = Select(t=w530, s=w531, f=w529) -> (s? t:f=w528:i32)
                  n195 = Array Subset(array=w551, index=w550, length=w528) -> (w549:refnum<class "Robot.lvclass">[])
                  n196 = property class="Robot"(reference=w542) -> (reference out=w537:refnum<class "Robot.lvclass">, "id"=w539:i32)  [unwired: 1 in, 1 out]
                  n197 = feedback #6(-1) -> (w541:i32)
                  n198 = Not Equal?(x=w539, y=w541) -> (x != y?=w538:bool)
                  n199 = feedback-in #6(w539) -> ()
                  n200 = Absolute Value(x=w561) -> (abs(x)=w565:dbl)
                  n201 = Absolute Value(x=w560) -> (abs(x)=w564:dbl)
                  n202 = Less Or Equal?(x=w564, y=0.1) -> (x <= y?=w562:bool)
                  n203 = Less Or Equal?(x=w565, y=0.1) -> (x <= y?=w563:bool)
                  n204 = Compound Arithmetic op=AND(w563, w562) -> (w558:bool)
                  n205 = Compound Arithmetic op=OR(w557, w558, w552) -> ()  [unwired: 1 out]
                  n206 = disable-structure shown="Enabled" {
                    disable-tunnel: w556 -> [w586 w664]
                    disable-tunnel: w555 -> [w585 w663]
                    disable-tunnel: [w584 w662] -> w554
                    disable-tunnel: w553 -> [w583 w668]
                    disable-tunnel: w549 -> [w582 w667]
                    disable-tunnel: w543 -> [w581 w665]
                    disable-tunnel: w538 -> [w580 _]
                    disable-tunnel: w537 -> [w579 w666]
                    disable-tunnel: w535 -> [_ w661]
                    frame Disabled {
                      n207 = case shown="True" w580 {
                        tunnel: w581 -> [_ _]
                        tunnel: w586 -> [w590 w632]
                        tunnel: w585 -> [_ w631]
                        tunnel: w582 -> [w593 w627]
                        tunnel: [w587 w625] -> w584
                        tunnel: w583 -> [w592 _]
                        tunnel: w579 -> [_ w619]
                        frame False {
                          n208 = property class="Ally"(reference=w592) -> ("RobotRef"=w591:refnum<class "Robot.lvclass">[])  [unwired: 1 in, 2 out]
                          n209 = for {
                            shift-right: [w595] -> w588
                            shift-left: w593 -> [w598]
                            shift-right: [w596] -> w589
                            shift-left: refnum<class "Robot.lvclass">[] [] -> [w599]
                            tunnel: w591 -> [w600] mode=indexing
                            tunnel: w590 -> [w597]
                            n210 = property class="Robot"(reference=w600) -> ("id"=w605:i32)  [unwired: 1 in, 2 out]
                            n211 = call "FindRobotByID.vi"("id"=w605, "RobotRef"=w598, "Utilities in"=w597) -> ("index"=w602:i32, "Robot"=w606:refnum<class "Robot.lvclass">, "Utilities out"=w604:refnum<class "Utilities.lvclass">)  [unwired: 5 in, 1 out]
                            n212 = Equal?(x=w602, y=-1) -> (x = y?=w603:bool)
                            n213 = case shown="False" w603 {
                              tunnel: w606 -> [w607 _]
                              tunnel: [w613 w615] -> w596
                              tunnel: w599 -> [w612 w615]
                              tunnel: w598 -> [w611 w614]
                              tunnel: w605 -> [w610 _]
                              tunnel: [w609 w614] -> w595
                              tunnel: w604 -> [w608 _]
                              tunnel: w600 -> [_ _]
                              frame False {
                                n214 = Insert Into Array(array=w612, new element=w607) -> (w613:refnum<class "Robot.lvclass">[])  [unwired: 1 in]
                                n215 = call "DeleteRobotByID.vi"("id"=w610, "RobotRef"=w611, "Utilities in"=w608) -> ("RobotRef out"=w609:refnum<class "Robot.lvclass">[])  [unwired: 6 in, 2 out]
                              }
                              frame True {
                              }
                            }
                          }
                          n216 = for {
                            shift-right: [w616] -> w587
                            shift-left: w589 -> [w618]
                            tunnel: w588 -> [w617] mode=indexing
                            n217 = Insert Into Array(array=w618, new element=w617) -> (w616:refnum<class "Robot.lvclass">[])  [unwired: 1 in]
                          }
                        }
                        frame True {
                          # "\"troca pesonalidade\""
                          # "coloca o nosso robô mais próximo do inimigo mais perto da bola no inicio do vetor"
                          n218 = for {
                            tunnel: w627 -> [w655] mode=indexing
                            tunnel: w619 -> [w654]
                            shift-right: [w645] -> w630
                            shift-left: -1 ("id") -> [w641]
                            shift-right: [w643] -> _
                            shift-left: inf -> [w640]
                            tunnel: w632 -> [w639]
                            n219 = property class="Robot"(reference=w654) -> ("x"=w651:dbl, "y"=w650:dbl)  [unwired: 1 in, 2 out]
                            n220 = property class="Robot"(reference=w655) -> ("id"=w644:i32, "x"=w653:dbl, "y"=w652:dbl)  [unwired: 1 in, 2 out]
                            n221 = Build Array(w651, w650) -> (w648:dbl[])
                            n222 = Build Array(w653, w652) -> (w649:dbl[])
                            n223 = Subtract(x=w649, y=w648) -> (x-y=w647:dbl[])
                            n224 = call "Module.vi"("2D vector"=w647, "Utilities in"=w639) -> ("Modulo"=w642:dbl)  [unwired: 7 in, 2 out]
                            n225 = Less?(x=w642, y=w640) -> (x < y?=w646:bool)
                            n226 = case shown="True" w646 {
                              tunnel: [w657 w659] -> w645
                              tunnel: w644 -> [_ w659]
                              tunnel: [w656 w658] -> w643
                              tunnel: w642 -> [_ w658]
                              tunnel: w641 -> [w657 _]
                              tunnel: w640 -> [w656 _]
                              frame False {
                              }
                              frame True {
                              }
                            }
                          }
                          n227 = call "FindRobotByID.vi"("id"=w630, "RobotRef"=w627, "Utilities in"=w631) -> ("index"=w622:i32, "Robot"=w628:refnum<class "Robot.lvclass">, "Utilities out"=w629:refnum<class "Utilities.lvclass">)  [unwired: 5 in, 1 out]
                          n228 = Not Equal?(x=-1, y=w622) -> (x != y?=w620:bool)
                          n229 = call "DeleteRobotByID.vi"("id"=w630, "RobotRef"=w627, "Utilities in"=w629) -> ("RobotRef out"=w624:refnum<class "Robot.lvclass">[])  [unwired: 6 in, 2 out]
                          n230 = case shown="False" w620 {
                            tunnel: w628 -> [_ w638]
                            tunnel: 0 ("index") -> [_ w637]
                            tunnel: [w634 w636] -> w625
                            tunnel: w624 -> [w634 w635]
                            frame False {
                            }
                            frame True {
                              n231 = Insert Into Array(array=w635, index=w637, new element=w638) -> (w636:refnum<class "Robot.lvclass">[])
                            }
                          }
                        }
                      }
                    }
                    frame Enabled {
                      n232 = case shown="True" TRUE {
                        tunnel: w665 -> [_ _]
                        tunnel: w664 -> [w672 w715]
                        tunnel: w663 -> [_ w714]
                        tunnel: w667 -> [w675 w710]
                        tunnel: [w669 w708] -> w662
                        tunnel: w668 -> [w674 _]
                        tunnel: w666 -> [_ _]
                        tunnel: w661 -> [_ w702]
                        frame False {
                          n233 = property class="Ally"(reference=w674) -> ("RobotRef"=w673:refnum<class "Robot.lvclass">[])  [unwired: 1 in, 2 out]
                          n234 = for {
                            shift-right: [w677] -> w670
                            shift-left: w675 -> [w680]
                            shift-right: [w678] -> w671
                            shift-left: refnum<class "Robot.lvclass">[] [] -> [w681]
                            tunnel: w673 -> [w682] mode=indexing
                            tunnel: w672 -> [w679]
                            n235 = property class="Robot"(reference=w682) -> ("id"=w687:i32)  [unwired: 1 in, 2 out]
                            n236 = call "FindRobotByID.vi"("id"=w687, "RobotRef"=w680, "Utilities in"=w679) -> ("index"=w684:i32, "Robot"=w688:refnum<class "Robot.lvclass">, "Utilities out"=w686:refnum<class "Utilities.lvclass">)  [unwired: 5 in, 1 out]
                            n237 = Equal?(x=w684, y=-1) -> (x = y?=w685:bool)
                            n238 = case shown="False" w685 {
                              tunnel: w688 -> [w689 _]
                              tunnel: [w695 w697] -> w678
                              tunnel: w681 -> [w694 w697]
                              tunnel: w680 -> [w693 w696]
                              tunnel: w687 -> [w692 _]
                              tunnel: [w691 w696] -> w677
                              tunnel: w686 -> [w690 _]
                              tunnel: w682 -> [_ _]
                              frame False {
                                n239 = Insert Into Array(array=w694, new element=w689) -> (w695:refnum<class "Robot.lvclass">[])  [unwired: 1 in]
                                n240 = call "DeleteRobotByID.vi"("id"=w692, "RobotRef"=w693, "Utilities in"=w690) -> ("RobotRef out"=w691:refnum<class "Robot.lvclass">[])  [unwired: 6 in, 2 out]
                              }
                              frame True {
                              }
                            }
                          }
                          n241 = for {
                            shift-right: [w698] -> w669
                            shift-left: w671 -> [w700]
                            tunnel: w670 -> [w699] mode=indexing
                            n242 = Insert Into Array(array=w700, new element=w699) -> (w698:refnum<class "Robot.lvclass">[])  [unwired: 1 in]
                          }
                        }
                        frame True {
                          # "Em vez do robo mais perto do inimigo mais perto da bola, pegamos simplesmente o mais proximo da bola"
                          # "\"troca pesonalidade\""
                          n243 = property class="Game"(reference=w702) -> ("BallRef"=w701:refnum<class "Ball.lvclass">)  [unwired: 1 in, 2 out]
                          n244 = for {
                            tunnel: w710 -> [w738] mode=indexing
                            tunnel: w701 -> [w737]
                            shift-right: [w728] -> w713
                            shift-left: -1 ("id") -> [w724]
                            shift-right: [w726] -> _
                            shift-left: inf -> [w723]
                            tunnel: w715 -> [w722]
                            n245 = property class="Robot"(reference=w738) -> ("id"=w727:i32, "x"=w736:dbl, "y"=w735:dbl)  [unwired: 1 in, 2 out]
                            n246 = property class="Ball"(reference=w737) -> ("x"=w734:dbl, "y"=w733:dbl)  [unwired: 1 in, 2 out]
                            n247 = Build Array(w734, w733) -> (w731:dbl[])
                            n248 = Build Array(w736, w735) -> (w732:dbl[])
                            n249 = Subtract(x=w732, y=w731) -> (x-y=w730:dbl[])
                            n250 = call "Module.vi"("2D vector"=w730, "Utilities in"=w722) -> ("Modulo"=w725:dbl)  [unwired: 7 in, 2 out]
                            n251 = Less?(x=w725, y=w723) -> (x < y?=w729:bool)
                            n252 = case shown="True" w729 {
                              tunnel: [w740 w742] -> w728
                              tunnel: w727 -> [_ w742]
                              tunnel: [w739 w741] -> w726
                              tunnel: w725 -> [_ w741]
                              tunnel: w724 -> [w740 _]
                              tunnel: w723 -> [w739 _]
                              frame False {
                              }
                              frame True {
                              }
                            }
                          }
                          n253 = call "FindRobotByID.vi"("id"=w713, "RobotRef"=w710, "Utilities in"=w714) -> ("index"=w705:i32, "Robot"=w711:refnum<class "Robot.lvclass">, "Utilities out"=w712:refnum<class "Utilities.lvclass">)  [unwired: 5 in, 1 out]
                          n254 = Not Equal?(x=-1, y=w705) -> (x != y?=w703:bool)
                          n255 = call "DeleteRobotByID.vi"("id"=w713, "RobotRef"=w710, "Utilities in"=w712) -> ("RobotRef out"=w707:refnum<class "Robot.lvclass">[])  [unwired: 6 in, 2 out]
                          n256 = case shown="False" w703 {
                            tunnel: w711 -> [_ w721]
                            tunnel: 0 ("index") -> [_ w720]
                            tunnel: [w717 w719] -> w708
                            tunnel: w707 -> [w717 w718]
                            frame False {
                            }
                            frame True {
                              n257 = Insert Into Array(array=w718, index=w720, new element=w721) -> (w719:refnum<class "Robot.lvclass">[])
                            }
                          }
                        }
                      }
                    }
                  }
                }
                frame Enabled {
                  n258 = Unbundle By Name(w769) -> ("AllyTeamArray"=w765:T4[], "maxDefendersNumber"=w762:i32)
                  n259 = call "newDangerEnemy.vi"("Game"=w750) -> ("numberOfPossible\nEnemiesToMark"=w751:i32)  [unwired: 11 in, 3 out]
                  n260 = Add(x=w751, y=1) -> (x+y=w749:i32)
                  n261 = call "PickActiveTeam.vi"("Robots"=w768, "AllyTeamArray"=w765, "Team"=AllyTeam."Attacker") -> ("Robots out"=w759:refnum<class "Robot.lvclass">[])  [unwired: 15 in, 1 out]
                  n262 = call "PickActiveTeam.vi"("Robots"=w768, "AllyTeamArray"=w765, "Team"=AllyTeam."Defender") -> ("Robots out"=w764:refnum<class "Robot.lvclass">[])  [unwired: 15 in, 1 out]
                  n263 = Array Size(array=w759) -> (size(s)=w758:i32)
                  n264 = Array Size(array=w764) -> (size(s)=w761:i32)
                  n265 = Subtract(x=w762, y=w761) -> (x-y=w755:i32)
                  n266 = Subtract(x=w758, y=w749) -> (x-y=w754:i32)
                  n267 = Build Array(0 ("y"), w755, w754) -> (w757:i32[])
                  n268 = Array Max & Min(array=w757) -> (max value=w753:i32)  [unwired: 3 out]
                  n269 = Delete From Array(array=w759, length=w753, index=0) -> (array with subset deleted=w743:refnum<class "Robot.lvclass">[])  [unwired: 1 out]
                  n270 = feedback #7(-1 ("y")) -> (w747:i32)
                  n271 = case shown="True" w744 {
                    tunnel: [w770 w773] -> w745
                    tunnel: w747 -> [w770 _]
                    tunnel: w746 -> [_ w772]
                    tunnel: w743 -> [_ w771]
                    frame False {
                    }
                    frame True {
                      n272 = call "findAllyOrEnemyRobotClosestToBall.vi"("Ally/Enemy Robots"=w771, "Ball"=w772) -> ("id"=w773:i32)  [unwired: 5 in, 4 out]
                    }
                  }
                  n273 = for {
                    tunnel: w743 -> [w782] mode=indexing
                    tunnel: w745 -> [w780]
                    tunnel: [w774] -> w760 mode=indexing
                    n274 = property class="Robot"(reference=w782) -> (reference out=w776:refnum<class "Robot.lvclass">, "id"=w781:i32)  [unwired: 1 in, 1 out]
                    n275 = Equal?(x=w781, y=w780) -> (x = y?=w779:bool)
                    n276 = Select(t=roles."AttackerBlock" ("role"), s=w779, f=roles."Marker" ("role")) -> (s? t:f=w775:T5)
                    n277 = property class="Robot"(reference=w776, "role"=w775) -> (reference out=w774:refnum<class "Robot.lvclass">)  [unwired: 1 in, 1 out]
                  }
                  n278 = feedback-in #7(w745) -> ()
                }
              }
            }
            frame "PrepareKickoffEnemy" {
              n279 = disable-structure shown="Enabled" {
                disable-tunnel: w801 -> [w835 _]
                disable-tunnel: w800 -> [w834 _]
                disable-tunnel: w799 -> [w831 _]
                disable-tunnel: w798 -> [w830 _]
                disable-tunnel: w797 -> [w829 _]
                disable-tunnel: [w828 w1020] -> w796
                disable-tunnel: w795 -> [w827 _]
                disable-tunnel: w794 -> [w826 _]
                disable-tunnel: w793 -> [w825 w1028]
                disable-tunnel: w792 -> [w824 _]
                disable-tunnel: w791 -> [w822 _]
                disable-tunnel: w790 -> [w821 _]
                disable-tunnel: w789 -> [w820 _]
                disable-tunnel: w788 -> [w819 _]
                disable-tunnel: w787 -> [w817 _]
                disable-tunnel: w786 -> [w809 _]
                disable-tunnel: w785 -> [w808 w1029]
                frame Disabled {
                  w804 = 1 ("y")
                  # "Deve trocar quem vai pra bola\nquando trocar robô inimigo mais\nperto da bola"
                  # "new offensive team"
                  # "True: bola parada e não está \nfora do campo. Não muda\nos robôs de ordem no vetor"
                  n280 = case shown="0" w821 {
                    tunnel: [0 ("number_of_robots") 1 w844 w851] -> w810
                    tunnel: w822 -> [_ _ w846 w850]
                    tunnel: w820 -> [_ _ w843 w849]
                    frame 0 {
                    }
                    frame 1..3 {
                    }
                    frame 4 {
                      n281 = Equal?(x=w846, y=2) -> (x = y?=w847:bool)
                      n282 = Decrement(x=w843) -> (x-1=w845:i32)
                      n283 = Select(t=w846, s=w847, f=w845) -> (s? t:f=w844:i32)
                    }
                    frame 5, 6, Default {
                      n284 = Less?(x=w849, y=w850) -> (x < y?=w852:bool)
                      n285 = Select(t=w849, s=w852, f=w850) -> (s? t:f=w851:i32)
                    }
                  }
                  n286 = Unbundle By Name(w808) -> ("Style"=w806:T9)
                  n287 = property class="Enemy"(reference=w819) -> ("RobotRef"=w818:refnum<class "Robot.lvclass">[])  [unwired: 1 in, 2 out]
                  n288 = call "filterNumberOfRobots.vi"("Game"=w809, "previousNumberOfRobots"=w810) -> ("finalNumberOfRobots"=w807:i32)  [unwired: 7 in, 2 out]
                  n289 = call "findAllyOrEnemyRobotClosestToBall.vi"("Ally/Enemy Robots"=w818, "Ball"=w817) -> ("Robot"=w816:refnum<class "Robot.lvclass">)  [unwired: 5 in, 4 out]
                  n290 = Subtract(x=w807, y=w806) -> (x-y=w803:i32)
                  n291 = Less Or Equal?(x=w803, y=w804) -> (x <= y?=w805:bool)
                  n292 = Select(t=w804, s=w805, f=w803) -> (s? t:f=w802:i32)
                  n293 = Array Subset(array=w825, index=w824, length=w802) -> (w823:refnum<class "Robot.lvclass">[])
                  n294 = property class="Robot"(reference=w816) -> (reference out=w811:refnum<class "Robot.lvclass">, "id"=w813:i32)  [unwired: 1 in, 1 out]
                  n295 = feedback #8(-1) -> (w815:i32)
                  n296 = Not Equal?(x=w813, y=w815) -> (x != y?=w812:bool)
                  n297 = feedback-in #8(w813) -> ()
                  n298 = Absolute Value(x=w835) -> (abs(x)=w839:dbl)
                  n299 = Absolute Value(x=w834) -> (abs(x)=w838:dbl)
                  n300 = Less Or Equal?(x=w838, y=0.1) -> (x <= y?=w836:bool)
                  n301 = Less Or Equal?(x=w839, y=0.1) -> (x <= y?=w837:bool)
                  n302 = Compound Arithmetic op=AND(w837, w836) -> (w832:bool)
                  n303 = Compound Arithmetic op=OR(w831, w832, w826) -> ()  [unwired: 1 out]
                  n304 = disable-structure shown="Enabled" {
                    disable-tunnel: w830 -> [w860 w938]
                    disable-tunnel: w829 -> [w859 w937]
                    disable-tunnel: [w858 w936] -> w828
                    disable-tunnel: w827 -> [w857 w942]
                    disable-tunnel: w823 -> [w856 w941]
                    disable-tunnel: w817 -> [w855 w939]
                    disable-tunnel: w812 -> [w854 _]
                    disable-tunnel: w811 -> [w853 w940]
                    disable-tunnel: w809 -> [_ w935]
                    frame Disabled {
                      n305 = case shown="True" w854 {
                        tunnel: w855 -> [_ _]
                        tunnel: w860 -> [w864 w906]
                        tunnel: w859 -> [_ w905]
                        tunnel: w856 -> [w867 w901]
                        tunnel: [w861 w899] -> w858
                        tunnel: w857 -> [w866 _]
                        tunnel: w853 -> [_ w893]
                        frame False {
                          n306 = property class="Ally"(reference=w866) -> ("RobotRef"=w865:refnum<class "Robot.lvclass">[])  [unwired: 1 in, 2 out]
                          n307 = for {
                            shift-right: [w869] -> w862
                            shift-left: w867 -> [w872]
                            shift-right: [w870] -> w863
                            shift-left: refnum<class "Robot.lvclass">[] [] -> [w873]
                            tunnel: w865 -> [w874] mode=indexing
                            tunnel: w864 -> [w871]
                            n308 = property class="Robot"(reference=w874) -> ("id"=w879:i32)  [unwired: 1 in, 2 out]
                            n309 = call "FindRobotByID.vi"("id"=w879, "RobotRef"=w872, "Utilities in"=w871) -> ("index"=w876:i32, "Robot"=w880:refnum<class "Robot.lvclass">, "Utilities out"=w878:refnum<class "Utilities.lvclass">)  [unwired: 5 in, 1 out]
                            n310 = Equal?(x=w876, y=-1) -> (x = y?=w877:bool)
                            n311 = case shown="False" w877 {
                              tunnel: w880 -> [w881 _]
                              tunnel: [w887 w889] -> w870
                              tunnel: w873 -> [w886 w889]
                              tunnel: w872 -> [w885 w888]
                              tunnel: w879 -> [w884 _]
                              tunnel: [w883 w888] -> w869
                              tunnel: w878 -> [w882 _]
                              tunnel: w874 -> [_ _]
                              frame False {
                                n312 = Insert Into Array(array=w886, new element=w881) -> (w887:refnum<class "Robot.lvclass">[])  [unwired: 1 in]
                                n313 = call "DeleteRobotByID.vi"("id"=w884, "RobotRef"=w885, "Utilities in"=w882) -> ("RobotRef out"=w883:refnum<class "Robot.lvclass">[])  [unwired: 6 in, 2 out]
                              }
                              frame True {
                              }
                            }
                          }
                          n314 = for {
                            shift-right: [w890] -> w861
                            shift-left: w863 -> [w892]
                            tunnel: w862 -> [w891] mode=indexing
                            n315 = Insert Into Array(array=w892, new element=w891) -> (w890:refnum<class "Robot.lvclass">[])  [unwired: 1 in]
                          }
                        }
                        frame True {
                          # "\"troca pesonalidade\""
                          # "coloca o nosso robô mais próximo do inimigo mais perto da bola no inicio do vetor"
                          n316 = for {
                            tunnel: w901 -> [w929] mode=indexing
                            tunnel: w893 -> [w928]
                            shift-right: [w919] -> w904
                            shift-left: -1 ("id") -> [w915]
                            shift-right: [w917] -> _
                            shift-left: inf -> [w914]
                            tunnel: w906 -> [w913]
                            n317 = property class="Robot"(reference=w928) -> ("x"=w925:dbl, "y"=w924:dbl)  [unwired: 1 in, 2 out]
                            n318 = property class="Robot"(reference=w929) -> ("id"=w918:i32, "x"=w927:dbl, "y"=w926:dbl)  [unwired: 1 in, 2 out]
                            n319 = Build Array(w925, w924) -> (w922:dbl[])
                            n320 = Build Array(w927, w926) -> (w923:dbl[])
                            n321 = Subtract(x=w923, y=w922) -> (x-y=w921:dbl[])
                            n322 = call "Module.vi"("2D vector"=w921, "Utilities in"=w913) -> ("Modulo"=w916:dbl)  [unwired: 7 in, 2 out]
                            n323 = Less?(x=w916, y=w914) -> (x < y?=w920:bool)
                            n324 = case shown="True" w920 {
                              tunnel: [w931 w933] -> w919
                              tunnel: w918 -> [_ w933]
                              tunnel: [w930 w932] -> w917
                              tunnel: w916 -> [_ w932]
                              tunnel: w915 -> [w931 _]
                              tunnel: w914 -> [w930 _]
                              frame False {
                              }
                              frame True {
                              }
                            }
                          }
                          n325 = call "FindRobotByID.vi"("id"=w904, "RobotRef"=w901, "Utilities in"=w905) -> ("index"=w896:i32, "Robot"=w902:refnum<class "Robot.lvclass">, "Utilities out"=w903:refnum<class "Utilities.lvclass">)  [unwired: 5 in, 1 out]
                          n326 = Not Equal?(x=-1, y=w896) -> (x != y?=w894:bool)
                          n327 = call "DeleteRobotByID.vi"("id"=w904, "RobotRef"=w901, "Utilities in"=w903) -> ("RobotRef out"=w898:refnum<class "Robot.lvclass">[])  [unwired: 6 in, 2 out]
                          n328 = case shown="False" w894 {
                            tunnel: w902 -> [_ w912]
                            tunnel: 0 ("index") -> [_ w911]
                            tunnel: [w908 w910] -> w899
                            tunnel: w898 -> [w908 w909]
                            frame False {
                            }
                            frame True {
                              n329 = Insert Into Array(array=w909, index=w911, new element=w912) -> (w910:refnum<class "Robot.lvclass">[])
                            }
                          }
                        }
                      }
                    }
                    frame Enabled {
                      n330 = case shown="True" TRUE {
                        tunnel: w939 -> [_ _]
                        tunnel: w938 -> [w946 w989]
                        tunnel: w937 -> [_ w988]
                        tunnel: w941 -> [w949 w984]
                        tunnel: [w943 w982] -> w936
                        tunnel: w942 -> [w948 _]
                        tunnel: w940 -> [_ _]
                        tunnel: w935 -> [_ w976]
                        frame False {
                          n331 = property class="Ally"(reference=w948) -> ("RobotRef"=w947:refnum<class "Robot.lvclass">[])  [unwired: 1 in, 2 out]
                          n332 = for {
                            shift-right: [w951] -> w944
                            shift-left: w949 -> [w954]
                            shift-right: [w952] -> w945
                            shift-left: refnum<class "Robot.lvclass">[] [] -> [w955]
                            tunnel: w947 -> [w956] mode=indexing
                            tunnel: w946 -> [w953]
                            n333 = property class="Robot"(reference=w956) -> ("id"=w961:i32)  [unwired: 1 in, 2 out]
                            n334 = call "FindRobotByID.vi"("id"=w961, "RobotRef"=w954, "Utilities in"=w953) -> ("index"=w958:i32, "Robot"=w962:refnum<class "Robot.lvclass">, "Utilities out"=w960:refnum<class "Utilities.lvclass">)  [unwired: 5 in, 1 out]
                            n335 = Equal?(x=w958, y=-1) -> (x = y?=w959:bool)
                            n336 = case shown="False" w959 {
                              tunnel: w962 -> [w963 _]
                              tunnel: [w969 w971] -> w952
                              tunnel: w955 -> [w968 w971]
                              tunnel: w954 -> [w967 w970]
                              tunnel: w961 -> [w966 _]
                              tunnel: [w965 w970] -> w951
                              tunnel: w960 -> [w964 _]
                              tunnel: w956 -> [_ _]
                              frame False {
                                n337 = Insert Into Array(array=w968, new element=w963) -> (w969:refnum<class "Robot.lvclass">[])  [unwired: 1 in]
                                n338 = call "DeleteRobotByID.vi"("id"=w966, "RobotRef"=w967, "Utilities in"=w964) -> ("RobotRef out"=w965:refnum<class "Robot.lvclass">[])  [unwired: 6 in, 2 out]
                              }
                              frame True {
                              }
                            }
                          }
                          n339 = for {
                            shift-right: [w972] -> w943
                            shift-left: w945 -> [w974]
                            tunnel: w944 -> [w973] mode=indexing
                            n340 = Insert Into Array(array=w974, new element=w973) -> (w972:refnum<class "Robot.lvclass">[])  [unwired: 1 in]
                          }
                        }
                        frame True {
                          # "Em vez do robo mais perto do inimigo mais perto da bola, pegamos simplesmente o mais proximo da bola"
                          # "\"troca pesonalidade\""
                          n341 = property class="Game"(reference=w976) -> ("BallRef"=w975:refnum<class "Ball.lvclass">)  [unwired: 1 in, 2 out]
                          n342 = for {
                            tunnel: w984 -> [w1012] mode=indexing
                            tunnel: w975 -> [w1011]
                            shift-right: [w1002] -> w987
                            shift-left: -1 ("id") -> [w998]
                            shift-right: [w1000] -> _
                            shift-left: inf -> [w997]
                            tunnel: w989 -> [w996]
                            n343 = property class="Robot"(reference=w1012) -> ("id"=w1001:i32, "x"=w1010:dbl, "y"=w1009:dbl)  [unwired: 1 in, 2 out]
                            n344 = property class="Ball"(reference=w1011) -> ("x"=w1008:dbl, "y"=w1007:dbl)  [unwired: 1 in, 2 out]
                            n345 = Build Array(w1008, w1007) -> (w1005:dbl[])
                            n346 = Build Array(w1010, w1009) -> (w1006:dbl[])
                            n347 = Subtract(x=w1006, y=w1005) -> (x-y=w1004:dbl[])
                            n348 = call "Module.vi"("2D vector"=w1004, "Utilities in"=w996) -> ("Modulo"=w999:dbl)  [unwired: 7 in, 2 out]
                            n349 = Less?(x=w999, y=w997) -> (x < y?=w1003:bool)
                            n350 = case shown="True" w1003 {
                              tunnel: [w1014 w1016] -> w1002
                              tunnel: w1001 -> [_ w1016]
                              tunnel: [w1013 w1015] -> w1000
                              tunnel: w999 -> [_ w1015]
                              tunnel: w998 -> [w1014 _]
                              tunnel: w997 -> [w1013 _]
                              frame False {
                              }
                              frame True {
                              }
                            }
                          }
                          n351 = call "FindRobotByID.vi"("id"=w987, "RobotRef"=w984, "Utilities in"=w988) -> ("index"=w979:i32, "Robot"=w985:refnum<class "Robot.lvclass">, "Utilities out"=w986:refnum<class "Utilities.lvclass">)  [unwired: 5 in, 1 out]
                          n352 = Not Equal?(x=-1, y=w979) -> (x != y?=w977:bool)
                          n353 = call "DeleteRobotByID.vi"("id"=w987, "RobotRef"=w984, "Utilities in"=w986) -> ("RobotRef out"=w981:refnum<class "Robot.lvclass">[])  [unwired: 6 in, 2 out]
                          n354 = case shown="False" w977 {
                            tunnel: w985 -> [_ w995]
                            tunnel: 0 ("index") -> [_ w994]
                            tunnel: [w991 w993] -> w982
                            tunnel: w981 -> [w991 w992]
                            frame False {
                            }
                            frame True {
                              n355 = Insert Into Array(array=w992, index=w994, new element=w995) -> (w993:refnum<class "Robot.lvclass">[])
                            }
                          }
                        }
                      }
                    }
                  }
                }
                frame Enabled {
                  n356 = Unbundle By Name(w1029) -> ("AllyTeamArray"=w1026:T4[])
                  n357 = call "PickActiveTeam.vi"("Robots"=w1028, "AllyTeamArray"=w1026, "Team"=AllyTeam."Attacker") -> ("Robots out"=w1019:refnum<class "Robot.lvclass">[])  [unwired: 15 in, 1 out]
                  n358 = Array Size(array=w1019) -> (size(s)=w1018:i32)
                  n359 = Subtract(x=w1018, y=2) -> (x-y=w1025:i32)
                  n360 = Max & Min(x=w1025, y=0) -> (max(x,y)=w1023:i32)  [unwired: 1 out]
                  n361 = Delete From Array(array=w1019, length=w1023, index=0) -> (array with subset deleted=w1021:refnum<class "Robot.lvclass">[])  [unwired: 1 out]
                  n362 = for {
                    tunnel: w1021 -> [w1037] mode=indexing
                    tunnel: [w1032] -> w1020 mode=indexing
                    i -> [w1031]
                    n363 = property class="Robot" props=["id"](reference=w1037) -> (reference out=w1034:refnum<class "Robot.lvclass">)  [unwired: 1 in, 2 out]
                    n364 = Equal To 0?(x=w1031) -> (x = 0?=w1030:bool)
                    n365 = Select(t=roles."AttackerBlock" ("role"), s=w1030, f=roles."FollowAttacker" ("role")) -> (s? t:f=w1033:T5)
                    n366 = property class="Robot"(reference=w1034, "role"=w1033) -> (reference out=w1032:refnum<class "Robot.lvclass">)  [unwired: 1 in, 1 out]
                  }
                }
              }
            }
            frame "PrepareKickoffAlly" {
              n367 = disable-structure shown="Enabled" {
                disable-tunnel: w1056 -> [w1090 _]
                disable-tunnel: w1055 -> [w1089 _]
                disable-tunnel: w1054 -> [w1086 _]
                disable-tunnel: w1053 -> [w1085 _]
                disable-tunnel: w1052 -> [w1084 _]
                disable-tunnel: [w1083 w1275] -> w1051
                disable-tunnel: w1050 -> [w1082 _]
                disable-tunnel: w1049 -> [w1081 _]
                disable-tunnel: w1048 -> [w1080 w1283]
                disable-tunnel: w1047 -> [w1079 _]
                disable-tunnel: w1046 -> [w1077 _]
                disable-tunnel: w1045 -> [w1076 _]
                disable-tunnel: w1044 -> [w1075 _]
                disable-tunnel: w1043 -> [w1074 _]
                disable-tunnel: w1042 -> [w1072 _]
                disable-tunnel: w1041 -> [w1064 _]
                disable-tunnel: w1040 -> [w1063 w1284]
                frame Disabled {
                  w1059 = 1 ("y")
                  # "Deve trocar quem vai pra bola\nquando trocar robô inimigo mais\nperto da bola"
                  # "new offensive team"
                  # "True: bola parada e não está \nfora do campo. Não muda\nos robôs de ordem no vetor"
                  n368 = case shown="0" w1076 {
                    tunnel: [0 ("number_of_robots") 1 w1099 w1106] -> w1065
                    tunnel: w1077 -> [_ _ w1101 w1105]
                    tunnel: w1075 -> [_ _ w1098 w1104]
                    frame 0 {
                    }
                    frame 1..3 {
                    }
                    frame 4 {
                      n369 = Equal?(x=w1101, y=2) -> (x = y?=w1102:bool)
                      n370 = Decrement(x=w1098) -> (x-1=w1100:i32)
                      n371 = Select(t=w1101, s=w1102, f=w1100) -> (s? t:f=w1099:i32)
                    }
                    frame 5, 6, Default {
                      n372 = Less?(x=w1104, y=w1105) -> (x < y?=w1107:bool)
                      n373 = Select(t=w1104, s=w1107, f=w1105) -> (s? t:f=w1106:i32)
                    }
                  }
                  n374 = Unbundle By Name(w1063) -> ("Style"=w1061:T9)
                  n375 = property class="Enemy"(reference=w1074) -> ("RobotRef"=w1073:refnum<class "Robot.lvclass">[])  [unwired: 1 in, 2 out]
                  n376 = call "filterNumberOfRobots.vi"("Game"=w1064, "previousNumberOfRobots"=w1065) -> ("finalNumberOfRobots"=w1062:i32)  [unwired: 7 in, 2 out]
                  n377 = call "findAllyOrEnemyRobotClosestToBall.vi"("Ally/Enemy Robots"=w1073, "Ball"=w1072) -> ("Robot"=w1071:refnum<class "Robot.lvclass">)  [unwired: 5 in, 4 out]
                  n378 = Subtract(x=w1062, y=w1061) -> (x-y=w1058:i32)
                  n379 = Less Or Equal?(x=w1058, y=w1059) -> (x <= y?=w1060:bool)
                  n380 = Select(t=w1059, s=w1060, f=w1058) -> (s? t:f=w1057:i32)
                  n381 = Array Subset(array=w1080, index=w1079, length=w1057) -> (w1078:refnum<class "Robot.lvclass">[])
                  n382 = property class="Robot"(reference=w1071) -> (reference out=w1066:refnum<class "Robot.lvclass">, "id"=w1068:i32)  [unwired: 1 in, 1 out]
                  n383 = feedback #9(-1) -> (w1070:i32)
                  n384 = Not Equal?(x=w1068, y=w1070) -> (x != y?=w1067:bool)
                  n385 = feedback-in #9(w1068) -> ()
                  n386 = Absolute Value(x=w1090) -> (abs(x)=w1094:dbl)
                  n387 = Absolute Value(x=w1089) -> (abs(x)=w1093:dbl)
                  n388 = Less Or Equal?(x=w1093, y=0.1) -> (x <= y?=w1091:bool)
                  n389 = Less Or Equal?(x=w1094, y=0.1) -> (x <= y?=w1092:bool)
                  n390 = Compound Arithmetic op=AND(w1092, w1091) -> (w1087:bool)
                  n391 = Compound Arithmetic op=OR(w1086, w1087, w1081) -> ()  [unwired: 1 out]
                  n392 = disable-structure shown="Enabled" {
                    disable-tunnel: w1085 -> [w1115 w1193]
                    disable-tunnel: w1084 -> [w1114 w1192]
                    disable-tunnel: [w1113 w1191] -> w1083
                    disable-tunnel: w1082 -> [w1112 w1197]
                    disable-tunnel: w1078 -> [w1111 w1196]
                    disable-tunnel: w1072 -> [w1110 w1194]
                    disable-tunnel: w1067 -> [w1109 _]
                    disable-tunnel: w1066 -> [w1108 w1195]
                    disable-tunnel: w1064 -> [_ w1190]
                    frame Disabled {
                      n393 = case shown="True" w1109 {
                        tunnel: w1110 -> [_ _]
                        tunnel: w1115 -> [w1119 w1161]
                        tunnel: w1114 -> [_ w1160]
                        tunnel: w1111 -> [w1122 w1156]
                        tunnel: [w1116 w1154] -> w1113
                        tunnel: w1112 -> [w1121 _]
                        tunnel: w1108 -> [_ w1148]
                        frame False {
                          n394 = property class="Ally"(reference=w1121) -> ("RobotRef"=w1120:refnum<class "Robot.lvclass">[])  [unwired: 1 in, 2 out]
                          n395 = for {
                            shift-right: [w1124] -> w1117
                            shift-left: w1122 -> [w1127]
                            shift-right: [w1125] -> w1118
                            shift-left: refnum<class "Robot.lvclass">[] [] -> [w1128]
                            tunnel: w1120 -> [w1129] mode=indexing
                            tunnel: w1119 -> [w1126]
                            n396 = property class="Robot"(reference=w1129) -> ("id"=w1134:i32)  [unwired: 1 in, 2 out]
                            n397 = call "FindRobotByID.vi"("id"=w1134, "RobotRef"=w1127, "Utilities in"=w1126) -> ("index"=w1131:i32, "Robot"=w1135:refnum<class "Robot.lvclass">, "Utilities out"=w1133:refnum<class "Utilities.lvclass">)  [unwired: 5 in, 1 out]
                            n398 = Equal?(x=w1131, y=-1) -> (x = y?=w1132:bool)
                            n399 = case shown="False" w1132 {
                              tunnel: w1135 -> [w1136 _]
                              tunnel: [w1142 w1144] -> w1125
                              tunnel: w1128 -> [w1141 w1144]
                              tunnel: w1127 -> [w1140 w1143]
                              tunnel: w1134 -> [w1139 _]
                              tunnel: [w1138 w1143] -> w1124
                              tunnel: w1133 -> [w1137 _]
                              tunnel: w1129 -> [_ _]
                              frame False {
                                n400 = Insert Into Array(array=w1141, new element=w1136) -> (w1142:refnum<class "Robot.lvclass">[])  [unwired: 1 in]
                                n401 = call "DeleteRobotByID.vi"("id"=w1139, "RobotRef"=w1140, "Utilities in"=w1137) -> ("RobotRef out"=w1138:refnum<class "Robot.lvclass">[])  [unwired: 6 in, 2 out]
                              }
                              frame True {
                              }
                            }
                          }
                          n402 = for {
                            shift-right: [w1145] -> w1116
                            shift-left: w1118 -> [w1147]
                            tunnel: w1117 -> [w1146] mode=indexing
                            n403 = Insert Into Array(array=w1147, new element=w1146) -> (w1145:refnum<class "Robot.lvclass">[])  [unwired: 1 in]
                          }
                        }
                        frame True {
                          # "\"troca pesonalidade\""
                          # "coloca o nosso robô mais próximo do inimigo mais perto da bola no inicio do vetor"
                          n404 = for {
                            tunnel: w1156 -> [w1184] mode=indexing
                            tunnel: w1148 -> [w1183]
                            shift-right: [w1174] -> w1159
                            shift-left: -1 ("id") -> [w1170]
                            shift-right: [w1172] -> _
                            shift-left: inf -> [w1169]
                            tunnel: w1161 -> [w1168]
                            n405 = property class="Robot"(reference=w1183) -> ("x"=w1180:dbl, "y"=w1179:dbl)  [unwired: 1 in, 2 out]
                            n406 = property class="Robot"(reference=w1184) -> ("id"=w1173:i32, "x"=w1182:dbl, "y"=w1181:dbl)  [unwired: 1 in, 2 out]
                            n407 = Build Array(w1180, w1179) -> (w1177:dbl[])
                            n408 = Build Array(w1182, w1181) -> (w1178:dbl[])
                            n409 = Subtract(x=w1178, y=w1177) -> (x-y=w1176:dbl[])
                            n410 = call "Module.vi"("2D vector"=w1176, "Utilities in"=w1168) -> ("Modulo"=w1171:dbl)  [unwired: 7 in, 2 out]
                            n411 = Less?(x=w1171, y=w1169) -> (x < y?=w1175:bool)
                            n412 = case shown="True" w1175 {
                              tunnel: [w1186 w1188] -> w1174
                              tunnel: w1173 -> [_ w1188]
                              tunnel: [w1185 w1187] -> w1172
                              tunnel: w1171 -> [_ w1187]
                              tunnel: w1170 -> [w1186 _]
                              tunnel: w1169 -> [w1185 _]
                              frame False {
                              }
                              frame True {
                              }
                            }
                          }
                          n413 = call "FindRobotByID.vi"("id"=w1159, "RobotRef"=w1156, "Utilities in"=w1160) -> ("index"=w1151:i32, "Robot"=w1157:refnum<class "Robot.lvclass">, "Utilities out"=w1158:refnum<class "Utilities.lvclass">)  [unwired: 5 in, 1 out]
                          n414 = Not Equal?(x=-1, y=w1151) -> (x != y?=w1149:bool)
                          n415 = call "DeleteRobotByID.vi"("id"=w1159, "RobotRef"=w1156, "Utilities in"=w1158) -> ("RobotRef out"=w1153:refnum<class "Robot.lvclass">[])  [unwired: 6 in, 2 out]
                          n416 = case shown="False" w1149 {
                            tunnel: w1157 -> [_ w1167]
                            tunnel: 0 ("index") -> [_ w1166]
                            tunnel: [w1163 w1165] -> w1154
                            tunnel: w1153 -> [w1163 w1164]
                            frame False {
                            }
                            frame True {
                              n417 = Insert Into Array(array=w1164, index=w1166, new element=w1167) -> (w1165:refnum<class "Robot.lvclass">[])
                            }
                          }
                        }
                      }
                    }
                    frame Enabled {
                      n418 = case shown="True" TRUE {
                        tunnel: w1194 -> [_ _]
                        tunnel: w1193 -> [w1201 w1244]
                        tunnel: w1192 -> [_ w1243]
                        tunnel: w1196 -> [w1204 w1239]
                        tunnel: [w1198 w1237] -> w1191
                        tunnel: w1197 -> [w1203 _]
                        tunnel: w1195 -> [_ _]
                        tunnel: w1190 -> [_ w1231]
                        frame False {
                          n419 = property class="Ally"(reference=w1203) -> ("RobotRef"=w1202:refnum<class "Robot.lvclass">[])  [unwired: 1 in, 2 out]
                          n420 = for {
                            shift-right: [w1206] -> w1199
                            shift-left: w1204 -> [w1209]
                            shift-right: [w1207] -> w1200
                            shift-left: refnum<class "Robot.lvclass">[] [] -> [w1210]
                            tunnel: w1202 -> [w1211] mode=indexing
                            tunnel: w1201 -> [w1208]
                            n421 = property class="Robot"(reference=w1211) -> ("id"=w1216:i32)  [unwired: 1 in, 2 out]
                            n422 = call "FindRobotByID.vi"("id"=w1216, "RobotRef"=w1209, "Utilities in"=w1208) -> ("index"=w1213:i32, "Robot"=w1217:refnum<class "Robot.lvclass">, "Utilities out"=w1215:refnum<class "Utilities.lvclass">)  [unwired: 5 in, 1 out]
                            n423 = Equal?(x=w1213, y=-1) -> (x = y?=w1214:bool)
                            n424 = case shown="False" w1214 {
                              tunnel: w1217 -> [w1218 _]
                              tunnel: [w1224 w1226] -> w1207
                              tunnel: w1210 -> [w1223 w1226]
                              tunnel: w1209 -> [w1222 w1225]
                              tunnel: w1216 -> [w1221 _]
                              tunnel: [w1220 w1225] -> w1206
                              tunnel: w1215 -> [w1219 _]
                              tunnel: w1211 -> [_ _]
                              frame False {
                                n425 = Insert Into Array(array=w1223, new element=w1218) -> (w1224:refnum<class "Robot.lvclass">[])  [unwired: 1 in]
                                n426 = call "DeleteRobotByID.vi"("id"=w1221, "RobotRef"=w1222, "Utilities in"=w1219) -> ("RobotRef out"=w1220:refnum<class "Robot.lvclass">[])  [unwired: 6 in, 2 out]
                              }
                              frame True {
                              }
                            }
                          }
                          n427 = for {
                            shift-right: [w1227] -> w1198
                            shift-left: w1200 -> [w1229]
                            tunnel: w1199 -> [w1228] mode=indexing
                            n428 = Insert Into Array(array=w1229, new element=w1228) -> (w1227:refnum<class "Robot.lvclass">[])  [unwired: 1 in]
                          }
                        }
                        frame True {
                          # "Em vez do robo mais perto do inimigo mais perto da bola, pegamos simplesmente o mais proximo da bola"
                          # "\"troca pesonalidade\""
                          n429 = property class="Game"(reference=w1231) -> ("BallRef"=w1230:refnum<class "Ball.lvclass">)  [unwired: 1 in, 2 out]
                          n430 = for {
                            tunnel: w1239 -> [w1267] mode=indexing
                            tunnel: w1230 -> [w1266]
                            shift-right: [w1257] -> w1242
                            shift-left: -1 ("id") -> [w1253]
                            shift-right: [w1255] -> _
                            shift-left: inf -> [w1252]
                            tunnel: w1244 -> [w1251]
                            n431 = property class="Robot"(reference=w1267) -> ("id"=w1256:i32, "x"=w1265:dbl, "y"=w1264:dbl)  [unwired: 1 in, 2 out]
                            n432 = property class="Ball"(reference=w1266) -> ("x"=w1263:dbl, "y"=w1262:dbl)  [unwired: 1 in, 2 out]
                            n433 = Build Array(w1263, w1262) -> (w1260:dbl[])
                            n434 = Build Array(w1265, w1264) -> (w1261:dbl[])
                            n435 = Subtract(x=w1261, y=w1260) -> (x-y=w1259:dbl[])
                            n436 = call "Module.vi"("2D vector"=w1259, "Utilities in"=w1251) -> ("Modulo"=w1254:dbl)  [unwired: 7 in, 2 out]
                            n437 = Less?(x=w1254, y=w1252) -> (x < y?=w1258:bool)
                            n438 = case shown="True" w1258 {
                              tunnel: [w1269 w1271] -> w1257
                              tunnel: w1256 -> [_ w1271]
                              tunnel: [w1268 w1270] -> w1255
                              tunnel: w1254 -> [_ w1270]
                              tunnel: w1253 -> [w1269 _]
                              tunnel: w1252 -> [w1268 _]
                              frame False {
                              }
                              frame True {
                              }
                            }
                          }
                          n439 = call "FindRobotByID.vi"("id"=w1242, "RobotRef"=w1239, "Utilities in"=w1243) -> ("index"=w1234:i32, "Robot"=w1240:refnum<class "Robot.lvclass">, "Utilities out"=w1241:refnum<class "Utilities.lvclass">)  [unwired: 5 in, 1 out]
                          n440 = Not Equal?(x=-1, y=w1234) -> (x != y?=w1232:bool)
                          n441 = call "DeleteRobotByID.vi"("id"=w1242, "RobotRef"=w1239, "Utilities in"=w1241) -> ("RobotRef out"=w1236:refnum<class "Robot.lvclass">[])  [unwired: 6 in, 2 out]
                          n442 = case shown="False" w1232 {
                            tunnel: w1240 -> [_ w1250]
                            tunnel: 0 ("index") -> [_ w1249]
                            tunnel: [w1246 w1248] -> w1237
                            tunnel: w1236 -> [w1246 w1247]
                            frame False {
                            }
                            frame True {
                              n443 = Insert Into Array(array=w1247, index=w1249, new element=w1250) -> (w1248:refnum<class "Robot.lvclass">[])
                            }
                          }
                        }
                      }
                    }
                  }
                }
                frame Enabled {
                  n444 = Unbundle By Name(w1284) -> ("AllyTeamArray"=w1281:T4[])
                  n445 = call "PickActiveTeam.vi"("Robots"=w1283, "AllyTeamArray"=w1281, "Team"=AllyTeam."Attacker") -> ("Robots out"=w1274:refnum<class "Robot.lvclass">[])  [unwired: 15 in, 1 out]
                  n446 = Array Size(array=w1274) -> (size(s)=w1273:i32)
                  n447 = Subtract(x=w1273, y=2) -> (x-y=w1280:i32)
                  n448 = Max & Min(x=w1280, y=0) -> (max(x,y)=w1278:i32)  [unwired: 1 out]
                  n449 = Delete From Array(array=w1274, length=w1278, index=0) -> (array with subset deleted=w1276:refnum<class "Robot.lvclass">[])  [unwired: 1 out]
                  n450 = for {
                    tunnel: w1276 -> [w1292] mode=indexing
                    tunnel: [w1287] -> w1275 mode=indexing
                    i -> [w1286]
                    n451 = property class="Robot" props=["id"](reference=w1292) -> (reference out=w1289:refnum<class "Robot.lvclass">)  [unwired: 1 in, 2 out]
                    n452 = Equal To 0?(x=w1286) -> (x = 0?=w1285:bool)
                    n453 = Select(t=roles."AttackerAimGoal" ("role"), s=w1285, f=roles."FollowAttacker" ("role")) -> (s? t:f=w1288:T5)
                    n454 = property class="Robot"(reference=w1289, "role"=w1288) -> (reference out=w1287:refnum<class "Robot.lvclass">)  [unwired: 1 in, 1 out]
                  }
                }
              }
            }
            frame "StopOffensive" {
              n455 = disable-structure shown="Enabled" {
                disable-tunnel: w1320 -> [w1380 _]
                disable-tunnel: w1319 -> [w1379 _]
                disable-tunnel: w1318 -> [w1376 _]
                disable-tunnel: w1317 -> [w1375 _]
                disable-tunnel: w1316 -> [w1374 _]
                disable-tunnel: [w1373 w1564] -> w1293
                disable-tunnel: w1315 -> [w1372 _]
                disable-tunnel: w1314 -> [w1371 _]
                disable-tunnel: w1313 -> [w1370 w1566]
                disable-tunnel: w1312 -> [w1369 _]
                disable-tunnel: w1311 -> [w1367 _]
                disable-tunnel: w1310 -> [w1366 _]
                disable-tunnel: w1309 -> [w1365 _]
                disable-tunnel: w1308 -> [w1364 _]
                disable-tunnel: w1307 -> [w1362 w1571]
                disable-tunnel: w1306 -> [w1354 w1567]
                disable-tunnel: w1305 -> [w1353 w1590]
                disable-tunnel: w1302 -> [_ w1573]
                disable-tunnel: w1301 -> [_ _]
                frame Disabled {
                  w1349 = 1 ("y")
                  # "Deve trocar quem vai pra bola\nquando trocar robô inimigo mais\nperto da bola"
                  # "new offensive team"
                  # "True: bola parada e não está \nfora do campo. Não muda\nos robôs de ordem no vetor"
                  n456 = case shown="0" w1366 {
                    tunnel: [0 ("number_of_robots") 1 w1389 w1396] -> w1355
                    tunnel: w1367 -> [_ _ w1391 w1395]
                    tunnel: w1365 -> [_ _ w1388 w1394]
                    frame 0 {
                    }
                    frame 1..3 {
                    }
                    frame 4 {
                      n457 = Equal?(x=w1391, y=2) -> (x = y?=w1392:bool)
                      n458 = Decrement(x=w1388) -> (x-1=w1390:i32)
                      n459 = Select(t=w1391, s=w1392, f=w1390) -> (s? t:f=w1389:i32)
                    }
                    frame 5, 6, Default {
                      n460 = Less?(x=w1394, y=w1395) -> (x < y?=w1397:bool)
                      n461 = Select(t=w1394, s=w1397, f=w1395) -> (s? t:f=w1396:i32)
                    }
                  }
                  n462 = Unbundle By Name(w1353) -> ("Style"=w1351:T9)
                  n463 = property class="Enemy"(reference=w1364) -> ("RobotRef"=w1363:refnum<class "Robot.lvclass">[])  [unwired: 1 in, 2 out]
                  n464 = call "filterNumberOfRobots.vi"("Game"=w1354, "previousNumberOfRobots"=w1355) -> ("finalNumberOfRobots"=w1352:i32)  [unwired: 7 in, 2 out]
                  n465 = call "findAllyOrEnemyRobotClosestToBall.vi"("Ally/Enemy Robots"=w1363, "Ball"=w1362) -> ("Robot"=w1361:refnum<class "Robot.lvclass">)  [unwired: 5 in, 4 out]
                  n466 = Subtract(x=w1352, y=w1351) -> (x-y=w1348:i32)
                  n467 = Less Or Equal?(x=w1348, y=w1349) -> (x <= y?=w1350:bool)
                  n468 = Select(t=w1349, s=w1350, f=w1348) -> (s? t:f=w1347:i32)
                  n469 = Array Subset(array=w1370, index=w1369, length=w1347) -> (w1368:refnum<class "Robot.lvclass">[])
                  n470 = property class="Robot"(reference=w1361) -> (reference out=w1356:refnum<class "Robot.lvclass">, "id"=w1358:i32)  [unwired: 1 in, 1 out]
                  n471 = feedback #10(-1) -> (w1360:i32)
                  n472 = Not Equal?(x=w1358, y=w1360) -> (x != y?=w1357:bool)
                  n473 = feedback-in #10(w1358) -> ()
                  n474 = Absolute Value(x=w1380) -> (abs(x)=w1384:dbl)
                  n475 = Absolute Value(x=w1379) -> (abs(x)=w1383:dbl)
                  n476 = Less Or Equal?(x=w1383, y=0.1) -> (x <= y?=w1381:bool)
                  n477 = Less Or Equal?(x=w1384, y=0.1) -> (x <= y?=w1382:bool)
                  n478 = Compound Arithmetic op=AND(w1382, w1381) -> (w1377:bool)
                  n479 = Compound Arithmetic op=OR(w1376, w1377, w1371) -> ()  [unwired: 1 out]
                  n480 = disable-structure shown="Enabled" {
                    disable-tunnel: w1375 -> [w1405 w1483]
                    disable-tunnel: w1374 -> [w1404 w1482]
                    disable-tunnel: [w1403 w1481] -> w1373
                    disable-tunnel: w1372 -> [w1402 w1487]
                    disable-tunnel: w1368 -> [w1401 w1486]
                    disable-tunnel: w1362 -> [w1400 w1484]
                    disable-tunnel: w1357 -> [w1399 _]
                    disable-tunnel: w1356 -> [w1398 w1485]
                    disable-tunnel: w1354 -> [_ w1480]
                    frame Disabled {
                      n481 = case shown="True" w1399 {
                        tunnel: w1400 -> [_ _]
                        tunnel: w1405 -> [w1409 w1451]
                        tunnel: w1404 -> [_ w1450]
                        tunnel: w1401 -> [w1412 w1446]
                        tunnel: [w1406 w1444] -> w1403
                        tunnel: w1402 -> [w1411 _]
                        tunnel: w1398 -> [_ w1438]
                        frame False {
                          n482 = property class="Ally"(reference=w1411) -> ("RobotRef"=w1410:refnum<class "Robot.lvclass">[])  [unwired: 1 in, 2 out]
                          n483 = for {
                            shift-right: [w1414] -> w1407
                            shift-left: w1412 -> [w1417]
                            shift-right: [w1415] -> w1408
                            shift-left: refnum<class "Robot.lvclass">[] [] -> [w1418]
                            tunnel: w1410 -> [w1419] mode=indexing
                            tunnel: w1409 -> [w1416]
                            n484 = property class="Robot"(reference=w1419) -> ("id"=w1424:i32)  [unwired: 1 in, 2 out]
                            n485 = call "FindRobotByID.vi"("id"=w1424, "RobotRef"=w1417, "Utilities in"=w1416) -> ("index"=w1421:i32, "Robot"=w1425:refnum<class "Robot.lvclass">, "Utilities out"=w1423:refnum<class "Utilities.lvclass">)  [unwired: 5 in, 1 out]
                            n486 = Equal?(x=w1421, y=-1) -> (x = y?=w1422:bool)
                            n487 = case shown="False" w1422 {
                              tunnel: w1425 -> [w1426 _]
                              tunnel: [w1432 w1434] -> w1415
                              tunnel: w1418 -> [w1431 w1434]
                              tunnel: w1417 -> [w1430 w1433]
                              tunnel: w1424 -> [w1429 _]
                              tunnel: [w1428 w1433] -> w1414
                              tunnel: w1423 -> [w1427 _]
                              tunnel: w1419 -> [_ _]
                              frame False {
                                n488 = Insert Into Array(array=w1431, new element=w1426) -> (w1432:refnum<class "Robot.lvclass">[])  [unwired: 1 in]
                                n489 = call "DeleteRobotByID.vi"("id"=w1429, "RobotRef"=w1430, "Utilities in"=w1427) -> ("RobotRef out"=w1428:refnum<class "Robot.lvclass">[])  [unwired: 6 in, 2 out]
                              }
                              frame True {
                              }
                            }
                          }
                          n490 = for {
                            shift-right: [w1435] -> w1406
                            shift-left: w1408 -> [w1437]
                            tunnel: w1407 -> [w1436] mode=indexing
                            n491 = Insert Into Array(array=w1437, new element=w1436) -> (w1435:refnum<class "Robot.lvclass">[])  [unwired: 1 in]
                          }
                        }
                        frame True {
                          # "\"troca pesonalidade\""
                          # "coloca o nosso robô mais próximo do inimigo mais perto da bola no inicio do vetor"
                          n492 = for {
                            tunnel: w1446 -> [w1474] mode=indexing
                            tunnel: w1438 -> [w1473]
                            shift-right: [w1464] -> w1449
                            shift-left: -1 ("id") -> [w1460]
                            shift-right: [w1462] -> _
                            shift-left: inf -> [w1459]
                            tunnel: w1451 -> [w1458]
                            n493 = property class="Robot"(reference=w1473) -> ("x"=w1470:dbl, "y"=w1469:dbl)  [unwired: 1 in, 2 out]
                            n494 = property class="Robot"(reference=w1474) -> ("id"=w1463:i32, "x"=w1472:dbl, "y"=w1471:dbl)  [unwired: 1 in, 2 out]
                            n495 = Build Array(w1470, w1469) -> (w1467:dbl[])
                            n496 = Build Array(w1472, w1471) -> (w1468:dbl[])
                            n497 = Subtract(x=w1468, y=w1467) -> (x-y=w1466:dbl[])
                            n498 = call "Module.vi"("2D vector"=w1466, "Utilities in"=w1458) -> ("Modulo"=w1461:dbl)  [unwired: 7 in, 2 out]
                            n499 = Less?(x=w1461, y=w1459) -> (x < y?=w1465:bool)
                            n500 = case shown="True" w1465 {
                              tunnel: [w1476 w1478] -> w1464
                              tunnel: w1463 -> [_ w1478]
                              tunnel: [w1475 w1477] -> w1462
                              tunnel: w1461 -> [_ w1477]
                              tunnel: w1460 -> [w1476 _]
                              tunnel: w1459 -> [w1475 _]
                              frame False {
                              }
                              frame True {
                              }
                            }
                          }
                          n501 = call "FindRobotByID.vi"("id"=w1449, "RobotRef"=w1446, "Utilities in"=w1450) -> ("index"=w1441:i32, "Robot"=w1447:refnum<class "Robot.lvclass">, "Utilities out"=w1448:refnum<class "Utilities.lvclass">)  [unwired: 5 in, 1 out]
                          n502 = Not Equal?(x=-1, y=w1441) -> (x != y?=w1439:bool)
                          n503 = call "DeleteRobotByID.vi"("id"=w1449, "RobotRef"=w1446, "Utilities in"=w1448) -> ("RobotRef out"=w1443:refnum<class "Robot.lvclass">[])  [unwired: 6 in, 2 out]
                          n504 = case shown="False" w1439 {
                            tunnel: w1447 -> [_ w1457]
                            tunnel: 0 ("index") -> [_ w1456]
                            tunnel: [w1453 w1455] -> w1444
                            tunnel: w1443 -> [w1453 w1454]
                            frame False {
                            }
                            frame True {
                              n505 = Insert Into Array(array=w1454, index=w1456, new element=w1457) -> (w1455:refnum<class "Robot.lvclass">[])
                            }
                          }
                        }
                      }
                    }
                    frame Enabled {
                      n506 = case shown="True" TRUE {
                        tunnel: w1484 -> [_ _]
                        tunnel: w1483 -> [w1491 w1534]
                        tunnel: w1482 -> [_ w1533]
                        tunnel: w1486 -> [w1494 w1529]
                        tunnel: [w1488 w1527] -> w1481
                        tunnel: w1487 -> [w1493 _]
                        tunnel: w1485 -> [_ _]
                        tunnel: w1480 -> [_ w1521]
                        frame False {
                          n507 = property class="Ally"(reference=w1493) -> ("RobotRef"=w1492:refnum<class "Robot.lvclass">[])  [unwired: 1 in, 2 out]
                          n508 = for {
                            shift-right: [w1496] -> w1489
                            shift-left: w1494 -> [w1499]
                            shift-right: [w1497] -> w1490
                            shift-left: refnum<class "Robot.lvclass">[] [] -> [w1500]
                            tunnel: w1492 -> [w1501] mode=indexing
                            tunnel: w1491 -> [w1498]
                            n509 = property class="Robot"(reference=w1501) -> ("id"=w1506:i32)  [unwired: 1 in, 2 out]
                            n510 = call "FindRobotByID.vi"("id"=w1506, "RobotRef"=w1499, "Utilities in"=w1498) -> ("index"=w1503:i32, "Robot"=w1507:refnum<class "Robot.lvclass">, "Utilities out"=w1505:refnum<class "Utilities.lvclass">)  [unwired: 5 in, 1 out]
                            n511 = Equal?(x=w1503, y=-1) -> (x = y?=w1504:bool)
                            n512 = case shown="False" w1504 {
                              tunnel: w1507 -> [w1508 _]
                              tunnel: [w1514 w1516] -> w1497
                              tunnel: w1500 -> [w1513 w1516]
                              tunnel: w1499 -> [w1512 w1515]
                              tunnel: w1506 -> [w1511 _]
                              tunnel: [w1510 w1515] -> w1496
                              tunnel: w1505 -> [w1509 _]
                              tunnel: w1501 -> [_ _]
                              frame False {
                                n513 = Insert Into Array(array=w1513, new element=w1508) -> (w1514:refnum<class "Robot.lvclass">[])  [unwired: 1 in]
                                n514 = call "DeleteRobotByID.vi"("id"=w1511, "RobotRef"=w1512, "Utilities in"=w1509) -> ("RobotRef out"=w1510:refnum<class "Robot.lvclass">[])  [unwired: 6 in, 2 out]
                              }
                              frame True {
                              }
                            }
                          }
                          n515 = for {
                            shift-right: [w1517] -> w1488
                            shift-left: w1490 -> [w1519]
                            tunnel: w1489 -> [w1518] mode=indexing
                            n516 = Insert Into Array(array=w1519, new element=w1518) -> (w1517:refnum<class "Robot.lvclass">[])  [unwired: 1 in]
                          }
                        }
                        frame True {
                          # "Em vez do robo mais perto do inimigo mais perto da bola, pegamos simplesmente o mais proximo da bola"
                          # "\"troca pesonalidade\""
                          n517 = property class="Game"(reference=w1521) -> ("BallRef"=w1520:refnum<class "Ball.lvclass">)  [unwired: 1 in, 2 out]
                          n518 = for {
                            tunnel: w1529 -> [w1557] mode=indexing
                            tunnel: w1520 -> [w1556]
                            shift-right: [w1547] -> w1532
                            shift-left: -1 ("id") -> [w1543]
                            shift-right: [w1545] -> _
                            shift-left: inf -> [w1542]
                            tunnel: w1534 -> [w1541]
                            n519 = property class="Robot"(reference=w1557) -> ("id"=w1546:i32, "x"=w1555:dbl, "y"=w1554:dbl)  [unwired: 1 in, 2 out]
                            n520 = property class="Ball"(reference=w1556) -> ("x"=w1553:dbl, "y"=w1552:dbl)  [unwired: 1 in, 2 out]
                            n521 = Build Array(w1553, w1552) -> (w1550:dbl[])
                            n522 = Build Array(w1555, w1554) -> (w1551:dbl[])
                            n523 = Subtract(x=w1551, y=w1550) -> (x-y=w1549:dbl[])
                            n524 = call "Module.vi"("2D vector"=w1549, "Utilities in"=w1541) -> ("Modulo"=w1544:dbl)  [unwired: 7 in, 2 out]
                            n525 = Less?(x=w1544, y=w1542) -> (x < y?=w1548:bool)
                            n526 = case shown="True" w1548 {
                              tunnel: [w1559 w1561] -> w1547
                              tunnel: w1546 -> [_ w1561]
                              tunnel: [w1558 w1560] -> w1545
                              tunnel: w1544 -> [_ w1560]
                              tunnel: w1543 -> [w1559 _]
                              tunnel: w1542 -> [w1558 _]
                              frame False {
                              }
                              frame True {
                              }
                            }
                          }
                          n527 = call "FindRobotByID.vi"("id"=w1532, "RobotRef"=w1529, "Utilities in"=w1533) -> ("index"=w1524:i32, "Robot"=w1530:refnum<class "Robot.lvclass">, "Utilities out"=w1531:refnum<class "Utilities.lvclass">)  [unwired: 5 in, 1 out]
                          n528 = Not Equal?(x=-1, y=w1524) -> (x != y?=w1522:bool)
                          n529 = call "DeleteRobotByID.vi"("id"=w1532, "RobotRef"=w1529, "Utilities in"=w1531) -> ("RobotRef out"=w1526:refnum<class "Robot.lvclass">[])  [unwired: 6 in, 2 out]
                          n530 = case shown="False" w1522 {
                            tunnel: w1530 -> [_ w1540]
                            tunnel: 0 ("index") -> [_ w1539]
                            tunnel: [w1536 w1538] -> w1527
                            tunnel: w1526 -> [w1536 w1537]
                            frame False {
                            }
                            frame True {
                              n531 = Insert Into Array(array=w1537, index=w1539, new element=w1540) -> (w1538:refnum<class "Robot.lvclass">[])
                            }
                          }
                        }
                      }
                    }
                  }
                }
                frame Enabled {
                  n532 = Unbundle By Name(w1590) -> ("AllyTeamArray"=w1587:T4[], "maxDefendersNumber"=w1584:i32)
                  n533 = call "newDangerEnemy.vi"("Game"=w1567) -> ("numberOfPossible\nEnemiesToMark"=w1568:i32)  [unwired: 11 in, 3 out]
                  n534 = call "PickActiveTeam.vi"("Robots"=w1566, "AllyTeamArray"=w1587, "Team"=AllyTeam."Attacker") -> ("Robots out"=w1563:refnum<class "Robot.lvclass">[])  [unwired: 15 in, 1 out]
                  n535 = call "PickActiveTeam.vi"("Robots"=w1566, "AllyTeamArray"=w1587, "Team"=AllyTeam."Defender") -> ("Robots out"=w1586:refnum<class "Robot.lvclass">[])  [unwired: 15 in, 1 out]
                  n536 = Array Size(array=w1563) -> (size(s)=w1577:i32)
                  n537 = Array Size(array=w1586) -> (size(s)=w1583:i32)
                  n538 = Add(x=w1568, y=1) -> (x+y=w1576:i32)
                  n539 = Subtract(x=w1577, y=w1576) -> (x-y=w1575:i32)
                  n540 = Subtract(x=w1584, y=w1583) -> (x-y=w1580:i32)
                  n541 = Build Array(0 ("y"), w1580, w1575) -> (w1579:i32[])
                  n542 = Array Max & Min(array=w1579) -> (max value=w1578:i32)  [unwired: 3 out]
                  n543 = Delete From Array(array=w1563, length=w1578, index=0) -> (deleted portion=w1562:refnum<class "Robot.lvclass">[], array with subset deleted=w1572:refnum<class "Robot.lvclass">[])
                  n544 = feedback #11(-1 ("y")) -> (w1569:i32)
                  n545 = case shown="True" w1573 {
                    tunnel: w1572 -> [_ w1594]
                    tunnel: w1571 -> [_ w1593]
                    tunnel: [w1591 w1592] -> w1570
                    tunnel: w1569 -> [w1591 _]
                    frame False {
                    }
                    frame True {
                      n546 = call "findAllyOrEnemyRobotClosestToBall.vi"("Ally/Enemy Robots"=w1594, "Ball"=w1593) -> ("id"=w1592:i32)  [unwired: 5 in, 4 out]
                    }
                  }
                  n547 = for {
                    tunnel: w1572 -> [w1603] mode=indexing
                    tunnel: w1570 -> [w1595]
                    tunnel: [w1596] -> w1565 mode=indexing
                    n548 = property class="Robot"(reference=w1603) -> (reference out=w1598:refnum<class "Robot.lvclass">, "id"=w1602:i32)  [unwired: 1 in, 1 out]
                    n549 = Equal?(x=w1602, y=w1595) -> (x = y?=w1601:bool)
                    n550 = Select(t=roles."AttackerStop" ("role"), s=w1601, f=roles."Marker" ("role")) -> (s? t:f=w1597:T5)
                    n551 = property class="Robot"(reference=w1598, "role"=w1597) -> (reference out=w1596:refnum<class "Robot.lvclass">)  [unwired: 1 in, 1 out]
                  }
                  n552 = feedback-in #11(w1570) -> ()
                  n553 = Build Array (concatenate)(w1562, w1565) -> (w1564:refnum<class "Robot.lvclass">[])
                }
              }
              n554 = call "FindRobotByID.vi"("id"=5, "RobotRef"=w1293) -> ("Robot"=w1297:refnum<class "Robot.lvclass">)  [unwired: 6 in, 3 out]
              n555 = Search 1D Array(1D array=w1293, element=w1297) -> (index of element=w1296:i32)  [unwired: 1 in]
              n556 = property class="Robot"(reference=w1297) -> (reference out=w1300:refnum<class "Robot.lvclass">, "role"=w1299:T5)  [unwired: 1 in, 1 out]
              n557 = Array Size(array=w1293) -> (size(s)=w1294:i32)
              n558 = for {
                N: w1294 -> [_]
                tunnel: w1293 -> [w1328]
                tunnel: w1293 -> [w1326]
                tunnel: w1300 -> [w1324]
                tunnel: w1299 -> [w1323]
                tunnel: w1296 -> [w1322]
                tunnel: [w1321] -> w1295
                i -> [w1325]
                w1329 = roles."AttackerStop" ("role")
                n559 = Index Array(array=w1328, index=w1325) -> (element=w1327:refnum<class "Robot.lvclass">)
                n560 = property class="Robot"(reference=w1327) -> (reference out=w1330:refnum<class "Robot.lvclass">, "role"=w1334:T5)  [unwired: 1 in, 1 out]
                n561 = Not Equal?(x=w1329, y=w1323) -> (x != y?=w1332:bool)
                n562 = Equal?(x=w1334, y=w1329) -> (x = y?=w1333:bool)
                n563 = And(x=w1333, y=w1332) -> (x .and. y?=w1331:bool)
                n564 = case shown="True" w1331 {
                  tunnel: w1330 -> [_ w1346]
                  tunnel: w1329 -> [_ w1343]
                  tunnel: w1326 -> [w1335 w1345]
                  tunnel: w1324 -> [_ w1344]
                  tunnel: w1325 -> [_ w1341]
                  tunnel: w1322 -> [_ w1338]
                  tunnel: [w1335 w1337] -> w1321
                  frame False {
                  }
                  frame True {
                    n565 = property class="Robot"(reference=w1346, "role"=roles."Marker") -> (reference out=w1342:refnum<class "Robot.lvclass">)  [unwired: 1 in, 1 out]
                    n566 = property class="Robot"(reference=w1344, "role"=w1343) -> (reference out=w1339:refnum<class "Robot.lvclass">)  [unwired: 1 in, 1 out]
                    n567 = Replace Array Subset(array=w1345, new element=w1342, index=w1341) -> (w1340:refnum<class "Robot.lvclass">[])
                    n568 = Replace Array Subset(array=w1340, new element=w1339, index=w1338) -> (w1337:refnum<class "Robot.lvclass">[])
                  }
                }
              }
            }
            frame "5RobotsNormalGamePlay" {
              n569 = disable-structure shown="Enabled" {
                disable-tunnel: w1620 -> [w1634 w1783]
                disable-tunnel: w1619 -> [w1633 _]
                disable-tunnel: w1618 -> [w1632 _]
                disable-tunnel: w1617 -> [w1631 _]
                disable-tunnel: w1616 -> [w1630 _]
                disable-tunnel: w1615 -> [w1629 w1775]
                disable-tunnel: w1614 -> [w1628 _]
                disable-tunnel: [w1627 w1780] -> w1613
                disable-tunnel: w1612 -> [w1624 w1779]
                disable-tunnel: w1611 -> [w1623 _]
                disable-tunnel: w1610 -> [w1622 _]
                disable-tunnel: w1609 -> [_ w1782]
                disable-tunnel: w1608 -> [w1621 w1765]
                disable-tunnel: w1607 -> [_ w1778]
                disable-tunnel: w1606 -> [_ w1777]
                disable-tunnel: [w1621 w1776] -> w1605
                frame Disabled {
                  # "new offensive team"
                  n570 = case shown="5, 6, Default" w1631 {
                    tunnel: [0 ("number_of_robots") 1 w1752 w1758] -> w1635
                    tunnel: w1630 -> [_ _ w1753 w1757]
                    tunnel: w1632 -> [_ _ w1749 w1756]
                    frame 0, 1 {
                    }
                    frame 2, 3 {
                    }
                    frame 4 {
                      n571 = Subtract(x=w1749, y=2) -> (x-y=w1750:i32)
                      n572 = Equal?(x=w1753, y=2) -> (x = y?=w1754:bool)
                      n573 = Select(t=w1753, s=w1754, f=w1750) -> (s? t:f=w1752:i32)
                    }
                    frame 5, 6, Default {
                      n574 = Less?(x=w1756, y=w1757) -> (x < y?=w1759:bool)
                      n575 = Select(t=w1756, s=w1759, f=w1757) -> (s? t:f=w1758:i32)
                    }
                  }
                  n576 = Array Subset(array=w1634, index=w1633, length=w1635) -> (w1626:refnum<class "Robot.lvclass">[])
                  n577 = Empty Array?(array=w1626) -> (empty?=w1625:bool)
                  n578 = case shown="False" w1625 {
                    tunnel: w1629 -> [w1650 _]
                    tunnel: w1626 -> [w1665 _]
                    tunnel: w1628 -> [w1663 _]
                    tunnel: [w1636 refnum<class "Robot.lvclass">[] []] -> w1627
                    tunnel: w1624 -> [w1645 _]
                    tunnel: w1623 -> [w1660 _]
                    tunnel: w1622 -> [w1658 _]
                    frame False {
                      n579 = property class="Game"(reference=w1645) -> ("FieldRef"=w1656:refnum<class "Field.lvclass">)  [unwired: 1 in, 2 out]
                      n580 = property class="Field"(reference=w1656) -> ("field_length"=w1655:i32)  [unwired: 1 in, 2 out]
                      n581 = property class="Ball"(reference=w1650) -> ("x"=w1649:dbl, "y"=w1652:dbl, "position(x,y)"=w1641:dbl[])  [unwired: 1 in, 2 out]
                      n582 = Divide(x=w1655, y=-6) -> (x/y=w1653:dbl)
                      n583 = Build Array(w1649, w1652) -> (w1651:dbl[])
                      n584 = Less?(x=w1649, y=w1653) -> (x < y?=w1647:bool)
                      n585 = Equal?(x=w1660, y=OffensivePlay."5PreparePassGame") -> (x = y?=w1648:bool)
                      n586 = And(x=w1648, y=w1647) -> (x .and. y?=w1646:bool)
                      n587 = Not(x=w1658) -> (.not. x?=w1657:bool)
                      n588 = feedback #12() -> (w1661:i32)  [unwired: 1 in]
                      n589 = case shown="True" w1646 {
                        tunnel: -1 ("id") -> [w1708 _]
                        tunnel: inf -> [w1707 _]
                        tunnel: w1665 -> [w1706 w1737]
                        tunnel: w1663 -> [w1705 w1736]
                        tunnel: [w1704 w1735] -> w1662
                        tunnel: w1661 -> [w1703 _]
                        tunnel: w1657 -> [w1702 _]
                        tunnel: w1651 -> [w1700 w1738]
                        tunnel: w1648 -> [w1699 _]
                        frame False {
                          n590 = And(x=w1699, y=w1702) -> (x .and. y?=w1701:bool)
                          n591 = case shown="False" w1701 {
                            tunnel: w1708 -> [w1714 _]
                            tunnel: w1707 -> [w1713 _]
                            tunnel: [w1712 w1733] -> w1704
                            tunnel: w1706 -> [w1711 _]
                            tunnel: w1705 -> [w1710 _]
                            tunnel: w1703 -> [_ w1733]
                            tunnel: w1700 -> [w1709 _]
                            frame False {
                              n592 = for {
                                tunnel: w1711 -> [w1728] mode=indexing
                                shift-right: [w1722] -> w1712
                                shift-left: w1714 -> [w1718]
                                shift-right: [w1720] -> _
                                shift-left: w1713 -> [w1717]
                                tunnel: w1710 -> [w1716]
                                tunnel: w1709 -> [w1715]
                                n593 = property class="Robot"(reference=w1728) -> ("id"=w1721:i32, "x"=w1727:dbl, "y"=w1726:dbl)  [unwired: 1 in, 2 out]
                                n594 = Build Array(w1727, w1726) -> (w1725:dbl[])
                                n595 = Subtract(x=w1725, y=w1715) -> (x-y=w1724:dbl[])
                                n596 = call "Module.vi"("2D vector"=w1724, "Utilities in"=w1716) -> ("Modulo"=w1719:dbl)  [unwired: 7 in, 2 out]
                                n597 = Less?(x=w1719, y=w1717) -> (x < y?=w1723:bool)
                                n598 = case shown="True" w1723 {
                                tunnel: [w1730 w1732] -> w1722
                                tunnel: w1721 -> [_ w1732]
                                tunnel: [w1729 w1731] -> w1720
                                tunnel: w1719 -> [_ w1731]
                                tunnel: w1718 -> [w1730 _]
                                tunnel: w1717 -> [w1729 _]
                                frame False {
                                }
                                frame True {
                                }
                                }
                              }
                            }
                            frame True {
                            }
                          }
                        }
                        frame True {
                          n599 = for {
                            tunnel: w1737 -> [w1743] mode=indexing
                            shift-right: [w1741] -> w1735
                            shift-left: 100 ("id") -> [w1739]
                            tunnel: w1736 -> [_]
                            tunnel: w1738 -> [_]
                            n600 = property class="Robot"(reference=w1743) -> ("id"=w1740:i32)  [unwired: 1 in, 2 out]
                            n601 = Greater?(x=w1739, y=w1740) -> (0:w1742:bool)
                            n602 = case shown="False" w1742 {
                              tunnel: [w1744 w1745] -> w1741
                              tunnel: w1740 -> [_ w1745]
                              tunnel: w1739 -> [w1744 _]
                              frame False {
                              }
                              frame True {
                              }
                            }
                          }
                        }
                      }
                      n603 = feedback-in #12(w1662) -> ()
                      n604 = call "DeleteRobotByID.vi"("id"=w1662, "RobotRef"=w1665, "Utilities in"=w1663) -> ("RobotRef out"=w1638:refnum<class "Robot.lvclass">[])  [unwired: 6 in, 2 out]
                      n605 = call "FindRobotByID.vi"("id"=w1662, "RobotRef"=w1665, "Utilities in"=w1663) -> ("Robot"=w1643:refnum<class "Robot.lvclass">)  [unwired: 5 in, 3 out]
                      n606 = Insert Into Array(array=refnum<class "Robot.lvclass">[] [], new element=w1643) -> (w1639:refnum<class "Robot.lvclass">[])  [unwired: 1 in]
                      n607 = call-dynamic "5RobotsPosition.vi"("Game"=w1645, "Utilities in"=w1663) -> ("5Positions"=w1644:dbl[][])  [unwired: 7 in, 2 out]
                      n608 = disable-structure shown="Enabled" {
                        disable-tunnel: w1644 -> [w1671 w1683]
                        disable-tunnel: [w1670 w1683] -> w1642
                        disable-tunnel: w1641 -> [w1668 _]
                        frame Disabled {
                          n609 = for {
                            tunnel: w1671 -> [w1676] mode=indexing
                            tunnel: w1668 -> [w1682]
                            tunnel: [w1677] -> w1675 mode=indexing
                            n610 = Subtract(x=w1676, y=w1682) -> (x-y=w1679:dbl[])
                            n611 = Index Array(array=w1676) -> (element #1=w1680:dbl, element #2=w1678:dbl)  [unwired: 2 in]
                            n612 = call "Modulo.vi"("2D vector"=w1679) -> ("Modulo"=w1681:dbl)  [unwired: 10 in]
                            n613 = Build Array(w1680, w1678, w1681) -> (w1677:dbl[])
                          }
                          n614 = call "Sort 2D Array.vim"("index"=2, "dimension to index (column)"=enum16{"column", "row"}."column", "2D array"=w1675) -> ("sorted 2D array"=w1672:dbl[][])  [unwired: 7 in, 1 out]
                          n615 = Delete From Array(array=w1672, index (row)=0) -> (array with subset deleted=w1670:dbl[][])  [unwired: 2 in, 1 out]
                        }
                        frame Enabled {
                        }
                      }
                      n616 = Insert Into Array(array=w1639, new element=w1638) -> (w1637:refnum<class "Robot.lvclass">[])  [unwired: 1 in]
                      n617 = for {
                        tunnel: w1642 -> [w1690]
                        tunnel: [w1692] -> w1636 mode=indexing
                        tunnel: w1645 -> [w1691]
                        tunnel: w1637 -> [w1687] mode=indexing
                        tunnel: refnum<class "5RobotsSkill.lvclass"> refnum ("5RobotsSkill in") -> [w1689]
                        i -> [w1684]
                        n618 = case shown="5, Default" w1684 {
                          tunnel: [roles."5Robots1st" ("role") roles."5Robots2nd" ("role") roles."5Robots3rd" ("role") roles."5Robots4th" ("role") roles."5Robots5th" ("role") roles."Shoot" ("role")] -> w1685
                          frame 1 {
                          }
                          frame 2 {
                          }
                          frame 3 {
                          }
                          frame 4 {
                          }
                          frame 5, Default {
                          }
                          frame 0 {
                          }
                        }
                        n619 = property class="Robot"(reference=w1687, "role"=w1685) -> (reference out=w1686:refnum<class "Robot.lvclass">)  [unwired: 1 in, 1 out]
                        n620 = call-dynamic "5RobotsSkill.vi"("Eliminate"=EliminateEnum."1", "id"=w1684, "5Positions"=w1690, "Robot In"=w1686, "Game in"=w1691, "5RobotsSkill in"=w1689) -> ("Robot out"=w1692:refnum<class "Robot.lvclass">)  [unwired: 3 in, 2 out]
                      }
                    }
                    frame True {
                    }
                  }
                }
                frame Enabled {
                  n621 = property class="Ally"(reference=w1765) -> ("currentBallZone"=w1764:T7)  [unwired: 1 in, 2 out]
                  n622 = Unbundle By Name(w1782) -> ("AllyTeamArray"=w1781:T4[])
                  n623 = disable-structure shown="Enabled" {
                    disable-tunnel: w1783 -> [w1807 w1808]
                    disable-tunnel: w1781 -> [w1806 _]
                    disable-tunnel: [w1804 w1808] -> w1774
                    frame Enabled {
                      n624 = call "PickActiveTeam.vi"("Robots"=w1807, "AllyTeamArray"=w1806, "Team"=AllyTeam."Attacker") -> ("Robots out"=w1804:refnum<class "Robot.lvclass">[])  [unwired: 15 in, 1 out]
                    }
                    frame Disabled {
                    }
                  }
                  n625 = call "findAllyOrEnemyRobotClosestToBall.vi"("Ally/Enemy Robots"=w1774, "Ball"=w1775) -> ("Robot distance to ball"=w1763:dbl, "id"=w1761:i32)  [unwired: 5 in, 3 out]
                  n626 = property class="Ally"(reference=w1778) -> ("RobotRef"=w1772:refnum<class "Robot.lvclass">[])  [unwired: 1 in, 2 out]
                  n627 = Array Size(array=w1774) -> (size(s)=w1771:i32)
                  n628 = call "UpdateZones.vi"("Old Robots"=w1772, "object in"=w1765) -> ("object out"=w1773:refnum<class "Ally.lvclass">)  [unwired: 8 in, 1 out]
                  n629 = call "ChooseZones.vi"("NumberOfAttackers"=w1771, "Game"=w1779, "object in"=w1773) -> ("Zones"=w1770:refnum<class "Zone.lvclass">[], "object out"=w1768:refnum<class "Ally.lvclass">)  [unwired: 6 in, 1 out]
                  n630 = Less?(x=w1763, y=500.0) -> (x < y?=w1760:bool)
                  n631 = for {
                    tunnel: w1774 -> [w1798] mode=indexing
                    tunnel: [w1797] -> w1780 mode=indexing
                    tunnel: w1770 -> [w1792] mode=indexing
                    tunnel: w1777 -> [w1791]
                    shift-right: [w1787] -> w1767
                    shift-left: zones."Size" ("Enum") -> [w1790]
                    tunnel: w1761 -> [w1786]
                    tunnel: w1760 -> [w1785]
                    n632 = call-dynamic "IsPointIntoBounds.vi"("Point"=w1791, "object in"=w1792) -> ("IntoBounds"=w1784:bool, "object out"=w1789:refnum<class "Zone.lvclass">)  [unwired: 7 in, 1 out]
                    n633 = case shown="False" w1785 {
                      tunnel: w1798 -> [_ w1803]
                      tunnel: [w1799 w1802] -> w1795
                      tunnel: w1786 -> [_ w1800]
                      tunnel: w1784 -> [w1799 _]
                      frame False {
                      }
                      frame True {
                        n634 = property class="Robot"(reference=w1803) -> ("id"=w1801:i32)  [unwired: 1 in, 2 out]
                        n635 = Equal?(x=w1801, y=w1800) -> (x = y?=w1802:bool)
                      }
                    }
                    n636 = property class="Zone.lvclass"(reference=w1789) -> ("ZoneIndex"=w1788:i32)  [unwired: 1 in, 2 out]
                    n637 = Select(t=roles."Shoot" ("role"), s=w1795, f=roles."5Robots1st" ("role")) -> (s? t:f=w1793:T5)
                    n638 = property class="Robot"(reference=w1798, "role"=w1793, "Zone"=w1792) -> (reference out=w1797:refnum<class "Robot.lvclass">)  [unwired: 1 in, 1 out]
                    n639 = Select(t=w1788, s=w1784, f=w1790) -> (s? t:f=w1787:i32)
                  }
                  n640 = feedback-in #13(w1767) -> ()
                  n641 = feedback #13() -> (w1766:i32)  [unwired: 1 in]
                  n642 = Not Equal?(x=w1764, y=w1766) -> ()  [unwired: 1 out]
                  n643 = property class="Ally"(reference=w1768, "currentBallZone"=w1767) -> (reference out=w1776:refnum<class "Ally.lvclass">)  [unwired: 1 in, 1 out]
                }
              }
            }
            frame "5PreparePassGame" {
              n644 = Unbundle By Name(w1820) -> ("AllyTeamArray"=w1815:T4[])
              n645 = disable-structure shown="Enabled" {
                disable-tunnel: w1823 -> [w1900 w1901]
                disable-tunnel: w1815 -> [w1899 _]
                disable-tunnel: [w1897 w1901] -> w1811
                frame Enabled {
                  n646 = call "PickActiveTeam.vi"("Robots"=w1900, "AllyTeamArray"=w1899, "Team"=AllyTeam."Attacker") -> ("Robots out"=w1897:refnum<class "Robot.lvclass">[])  [unwired: 15 in, 1 out]
                }
                frame Disabled {
                }
              }
              n647 = call "findAllyOrEnemyRobotClosestToBall.vi"("Ally/Enemy Robots"=w1811, "Ball"=w1810) -> ("id"=w1809:i32)  [unwired: 5 in, 4 out]
              n648 = case shown="True" TRUE {
                tunnel: [w1838 w1874] -> w1822
                tunnel: w1821 -> [w1826 w1871]
                tunnel: w1811 -> [w1825 w1869]
                tunnel: w1810 -> [_ w1868]
                tunnel: w1819 -> [w1836 w1866]
                tunnel: w1818 -> [w1835 _]
                tunnel: w1817 -> [w1831 _]
                tunnel: [w1828 w1866] -> w1816
                tunnel: [w1824 w1865] -> w1813
                tunnel: w1812 -> [_ w1865]
                tunnel: w1809 -> [w1824 _]
                frame True {
                  n649 = property class="Ally"(reference=w1835) -> ("RobotRef"=w1834:refnum<class "Robot.lvclass">[])  [unwired: 1 in, 2 out]
                  n650 = Array Size(array=w1825) -> (size(s)=w1833:i32)
                  n651 = call "UpdateZones.vi"("Old Robots"=w1834, "object in"=w1836) -> ("object out"=w1837:refnum<class "Ally.lvclass">)  [unwired: 8 in, 1 out]
                  n652 = call "ChooseZones.vi"("NumberOfAttackers"=w1833, "Game"=w1826, "object in"=w1837) -> ("Zones"=w1832:refnum<class "Zone.lvclass">[], "object out"=w1829:refnum<class "Ally.lvclass">)  [unwired: 6 in, 1 out]
                  n653 = for {
                    tunnel: w1825 -> [w1847] mode=indexing
                    tunnel: [w1850] -> w1838 mode=indexing
                    tunnel: w1832 -> [w1840] mode=indexing
                    tunnel: w1831 -> [w1839]
                    shift-right: [w1843] -> w1827
                    shift-left: zones."Size" ("Enum") -> [w1842]
                    tunnel: w1826 -> [w1848]
                    tunnel: w1824 -> [w1846]
                    n654 = property class="Robot"(reference=w1847) -> ("id"=w1841:i32)  [unwired: 1 in, 2 out]
                    n655 = Equal?(x=w1841, y=w1846) -> (x = y?=w1849:bool)
                    n656 = case shown="False" w1849 {
                      tunnel: w1847 -> [w1856 w1864]
                      tunnel: [w1854 w1863] -> w1850
                      tunnel: w1840 -> [w1853 w1861]
                      tunnel: w1848 -> [w1852 _]
                      frame False {
                        n657 = disable-structure shown="Enabled" {
                          disable-tunnel: w1853 -> [w1859 w1860]
                          disable-tunnel: w1852 -> [w1858 _]
                          disable-tunnel: [w1857 w1860] -> w1851
                          frame Enabled {
                            n658 = call "SearchTarget.vi"("Game"=w1858, "object in"=w1859) -> ("object out"=w1857:refnum<class "Zone.lvclass">)  [unwired: 8 in, 1 out]
                          }
                          frame Disabled {
                          }
                        }
                        n659 = property class="Robot"(reference=w1856, "role"=roles."5Robots1st", "Zone"=w1851) -> (reference out=w1854:refnum<class "Robot.lvclass">)  [unwired: 1 in, 1 out]
                      }
                      frame True {
                        n660 = property class="Robot"(reference=w1864, "role"=roles."AttackerStop", "Zone"=w1861) -> (reference out=w1863:refnum<class "Robot.lvclass">)  [unwired: 1 in, 1 out]
                      }
                    }
                    n661 = property class="Zone.lvclass"(reference=w1840) -> ("ZoneIndex"=w1844:i32)  [unwired: 1 in, 2 out]
                    n662 = call-dynamic "IsPointIntoBounds.vi"("Point"=w1839, "object in"=w1840) -> ("IntoBounds"=w1845:bool)  [unwired: 7 in, 2 out]
                    n663 = Select(t=w1844, s=w1845, f=w1842) -> (s? t:f=w1843:i32)
                  }
                  n664 = property class="Ally"(reference=w1829, "currentBallZone"=w1827) -> (reference out=w1828:refnum<class "Ally.lvclass">)  [unwired: 1 in, 1 out]
                }
                frame False {
                  n665 = call "findAllyOrEnemyRobotClosestToBall.vi"("Ally/Enemy Robots"=w1869, "Ball"=w1868) -> ("id"=w1867:i32)  [unwired: 5 in, 4 out]
                  n666 = call-dynamic "5RobotsPosition.vi"("Game"=w1871, "Utilities in"=refnum<class "Utilities.lvclass"> refnum) -> ("5Positions"=w1870:dbl[][])  [unwired: 7 in, 2 out]
                  n667 = for {
                    tunnel: w1869 -> [w1881] mode=indexing
                    tunnel: [w1875] -> w1874 mode=indexing
                    tunnel: refnum<class "5RobotsSkill.lvclass"> refnum ("5RobotsSkill in") -> [w1876]
                    tunnel: w1871 -> [w1877]
                    tunnel: w1870 -> [w1878]
                    tunnel: w1867 -> [w1883]
                    i -> [w1879]
                    n668 = property class="Robot"(reference=w1881) -> ("id"=w1884:i32)  [unwired: 1 in, 2 out]
                    n669 = Equal?(x=w1884, y=w1883) -> (x = y?=w1882:bool)
                    n670 = case shown="False" w1882 {
                      tunnel: w1881 -> [w1893 w1896]
                      tunnel: EliminateEnum."1" ("Eliminate") -> [w1891 _]
                      tunnel: w1879 -> [w1890 _]
                      tunnel: w1878 -> [w1889 _]
                      tunnel: w1877 -> [w1887 _]
                      tunnel: w1876 -> [w1886 _]
                      tunnel: [w1885 w1895] -> w1875
                      frame False {
                        n671 = property class="Robot"(reference=w1893, "role"=roles."5Robots1st") -> (reference out=w1888:refnum<class "Robot.lvclass">)  [unwired: 1 in, 1 out]
                        n672 = call-dynamic "5RobotsSkill.vi"("Eliminate"=w1891, "id"=w1890, "5Positions"=w1889, "Robot In"=w1888, "Game in"=w1887, "5RobotsSkill in"=w1886) -> ("Robot out"=w1885:refnum<class "Robot.lvclass">)  [unwired: 3 in, 2 out]
                      }
                      frame True {
                        n673 = property class="Robot"(reference=w1896, "role"=roles."AttackerStop" ("t")) -> (reference out=w1895:refnum<class "Robot.lvclass">)  [unwired: 1 in, 1 out]
                      }
                    }
                  }
                }
              }
            }
            frame "5RobotsPassGamePlay" {
              n674 = Unbundle By Name(w1910) -> ("AllyTeamArray"=w1905:T4[])
              n675 = disable-structure shown="Enabled" {
                disable-tunnel: w1914 -> [w2003 w2004]
                disable-tunnel: w1905 -> [w2002 _]
                disable-tunnel: [w2000 w2004] -> w1904
                frame Enabled {
                  n676 = call "PickActiveTeam.vi"("Robots"=w2003, "AllyTeamArray"=w2002, "Team"=AllyTeam."Attacker") -> ("Robots out"=w2000:refnum<class "Robot.lvclass">[])  [unwired: 15 in, 1 out]
                }
                frame Disabled {
                }
              }
              n677 = case shown="True" TRUE {
                tunnel: [w1934 w1977] -> w1912
                tunnel: w1911 -> [w1924 w1974]
                tunnel: w1904 -> [w1923 w1972]
                tunnel: w1913 -> [_ w1971]
                tunnel: w1909 -> [w1932 w1969]
                tunnel: w1908 -> [w1931 _]
                tunnel: w1907 -> [w1915 _]
                tunnel: [w1926 w1969] -> w1906
                tunnel: w1902 -> [w1916 _]
                frame True {
                  n678 = property class="Ally"(reference=w1931) -> ("RobotRef"=w1930:refnum<class "Robot.lvclass">[])  [unwired: 1 in, 2 out]
                  n679 = Array Size(array=w1923) -> (size(s)=w1929:i32)
                  n680 = call "UpdateZones.vi"("Old Robots"=w1930, "object in"=w1932) -> ("object out"=w1933:refnum<class "Ally.lvclass">)  [unwired: 8 in, 1 out]
                  n681 = call "ChooseZones.vi"("NumberOfAttackers"=w1929, "Game"=w1924, "object in"=w1933) -> ("Zones"=w1920:refnum<class "Zone.lvclass">[], "object out"=w1927:refnum<class "Ally.lvclass">)  [unwired: 6 in, 1 out]
                  n682 = for {
                    tunnel: w1923 -> [w1948] mode=indexing
                    tunnel: [w1945] -> w1922 mode=indexing
                    shift-right: [w1946] -> _
                    shift-left: 0.0 -> [w1940]
                    tunnel: w1920 -> [w1944] mode=indexing
                    tunnel: [w1943] -> w1919 mode=indexing
                    shift-right: [w1942] -> w1917
                    shift-left: -1 -> [w1947]
                    tunnel: w1916 -> [w1935]
                    n683 = property class="Robot"(reference=w1948) -> (reference out=w1945:refnum<class "Robot.lvclass">, "id"=w1936:i32)  [unwired: 1 in, 1 out]
                    n684 = property class="Zone.lvclass"(reference=w1944) -> (reference out=w1943:refnum<class "Zone.lvclass">, "targetEvaluation"=w1941:dbl)  [unwired: 1 in, 1 out]
                    n685 = Greater Or Equal?(x=w1941, y=w1940) -> (x >= y?=w1939:bool)
                    n686 = Not Equal?(x=w1936, y=w1935) -> (x != y?=w1937:bool)
                    n687 = And(x=w1939, y=w1937) -> (x .and. y?=w1938:bool)
                    n688 = Select(t=w1941, s=w1938, f=w1940) -> (s? t:f=w1946:dbl)
                    n689 = Select(t=w1936, s=w1938, f=w1947) -> (s? t:f=w1942:i32)
                  }
                  n690 = for {
                    tunnel: w1922 -> [w1967] mode=indexing
                    tunnel: [w1968] -> w1934 mode=indexing
                    tunnel: w1919 -> [w1954] mode=indexing
                    shift-right: [w1949] -> w1925
                    shift-left: zones."Size" ("Enum") -> [w1950]
                    tunnel: w1916 -> [w1966]
                    tunnel: w1917 -> [w1959]
                    tunnel: w1915 -> [w1955]
                    n691 = property class="Robot"(reference=w1967) -> (reference out=w1956:refnum<class "Robot.lvclass">, "id"=w1960:i32)  [unwired: 1 in, 1 out]
                    n692 = Equal?(x=w1960, y=w1966) -> (x = y?=w1965:bool)
                    n693 = Equal?(x=w1960, y=w1959) -> (x = y?=w1961:bool)
                    n694 = Select(t=roles."PassBestReceiver" ("role"), s=w1961, f=roles."5Robots1st") -> (s? t:f=w1962:T5)
                    n695 = Select(t=roles."PassBestRobot" ("role"), s=w1965, f=w1962) -> (s? t:f=w1963:T5)
                    n696 = call-dynamic "IsPointIntoBounds.vi"("Point"=w1955, "object in"=w1954) -> ("IntoBounds"=w1951:bool, "object out"=w1953:refnum<class "Zone.lvclass">)  [unwired: 7 in, 1 out]
                    n697 = property class="Zone.lvclass"(reference=w1953) -> ("ZoneIndex"=w1952:i32)  [unwired: 1 in, 2 out]
                    n698 = property class="Robot"(reference=w1956, "role"=w1963, "Zone"=w1954) -> (reference out=w1968:refnum<class "Robot.lvclass">)  [unwired: 1 in, 1 out]
                    n699 = Select(t=w1952, s=w1951, f=w1950) -> (s? t:f=w1949:i32)
                  }
                  n700 = property class="Ally"(reference=w1927, "currentBallZone"=w1925) -> (reference out=w1926:refnum<class "Ally.lvclass">)  [unwired: 1 in, 1 out]
                }
                frame False {
                  n701 = call "findAllyOrEnemyRobotClosestToBall.vi"("Ally/Enemy Robots"=w1972, "Ball"=w1971) -> ("id"=w1970:i32)  [unwired: 5 in, 4 out]
                  n702 = call-dynamic "5RobotsPosition.vi"("Game"=w1974, "Utilities in"=refnum<class "Utilities.lvclass"> refnum) -> ("5Positions"=w1973:dbl[][])  [unwired: 7 in, 2 out]
                  n703 = for {
                    tunnel: w1972 -> [w1984] mode=indexing
                    tunnel: [w1978] -> w1977 mode=indexing
                    tunnel: refnum<class "5RobotsSkill.lvclass"> refnum ("5RobotsSkill in") -> [w1979]
                    tunnel: w1974 -> [w1980]
                    tunnel: w1973 -> [w1981]
                    tunnel: w1970 -> [w1986]
                    i -> [w1982]
                    n704 = property class="Robot"(reference=w1984) -> ("id"=w1987:i32)  [unwired: 1 in, 2 out]
                    n705 = Equal?(x=w1987, y=w1986) -> (x = y?=w1985:bool)
                    n706 = case shown="False" w1985 {
                      tunnel: w1984 -> [w1996 w1999]
                      tunnel: EliminateEnum."1" ("Eliminate") -> [w1994 _]
                      tunnel: w1982 -> [w1993 _]
                      tunnel: w1981 -> [w1992 _]
                      tunnel: w1980 -> [w1990 _]
                      tunnel: w1979 -> [w1989 _]
                      tunnel: [w1988 w1998] -> w1978
                      frame False {
                        n707 = property class="Robot"(reference=w1996, "role"=roles."5Robots1st") -> (reference out=w1991:refnum<class "Robot.lvclass">)  [unwired: 1 in, 1 out]
                        n708 = call-dynamic "5RobotsSkill.vi"("Eliminate"=w1994, "id"=w1993, "5Positions"=w1992, "Robot In"=w1991, "Game in"=w1990, "5RobotsSkill in"=w1989) -> ("Robot out"=w1988:refnum<class "Robot.lvclass">)  [unwired: 3 in, 2 out]
                      }
                      frame True {
                        n709 = property class="Robot"(reference=w1999, "role"=roles."AttackerStop" ("t")) -> (reference out=w1998:refnum<class "Robot.lvclass">)  [unwired: 1 in, 1 out]
                      }
                    }
                  }
                }
              }
            }
            frame "Prepare Penalty Enemy", "PreparePenaltyAlly" {
              n710 = Unbundle By Name(w2018) -> ("AllyTeamArray"=w2017:T4[], "ShootOutRobotId"=w2012:dbl)
              n711 = call "PickActiveTeam.vi"("Robots"=w2019, "AllyTeamArray"=w2017, "Team"=AllyTeam."Attacker") -> ("Robots out"=w2014:refnum<class "Robot.lvclass">[])  [unwired: 15 in, 1 out]
              n712 = call "PickActiveTeam.vi"("Robots"=w2019, "AllyTeamArray"=w2017, "Team"=AllyTeam."Defender") -> ("Robots out"=w2020:refnum<class "Robot.lvclass">[])  [unwired: 15 in, 1 out]
              n713 = Insert Into Array(array=w2014, new element=w2020) -> (w2013:refnum<class "Robot.lvclass">[])  [unwired: 1 in]
              n714 = for {
                tunnel: w2013 -> [w2066] mode=indexing
                tunnel: w2012 -> [w2064]
                tunnel: [w2061] -> w2006 mode=indexing
                tunnel: w2011 -> [w2060]
                shift-right: [w2050] -> w2007
                shift-left: FALSE -> [w2053]
                n715 = property class="Robot"(reference=w2066) -> (reference out=w2062:refnum<class "Robot.lvclass">, "id"=w2065:i32)  [unwired: 1 in, 1 out]
                n716 = To Long Integer(number=w2064) -> (32bit integer=w2063:i32)
                n717 = Equal?(x=w2060, y=OffensivePlay."PreparePenaltyAlly") -> (x = y?=w2058:bool)
                n718 = Equal?(x=w2065, y=w2063) -> (x = y?=w2052:bool)
                n719 = And(x=w2052, y=w2058) -> (x .and. y?=w2057:bool)
                n720 = Select(t=roles."AttackerAimGoal" ("role"), s=w2057, f=roles."PenaltyDefense" ("role")) -> (s? t:f=w2054:T5)
                n721 = property class="Robot"(reference=w2062, "role"=w2054) -> (reference out=w2061:refnum<class "Robot.lvclass">)  [unwired: 1 in, 1 out]
                n722 = Select(t=TRUE, s=w2052, f=w2053) -> (s? t:f=w2050:bool)
              }
              n723 = case shown="False" w2007 {
                tunnel: w2006 -> [w2022 w2049]
                tunnel: [w2021 w2049] -> w2005
                frame False {
                  n724 = for {
                    N: 6 -> [_]
                    tunnel: w2022 -> [w2045]
                    tunnel: [w2044] -> w2023
                    i -> [w2043]
                    stop <- w2046 stop-if-true
                    n725 = Subtract(x=5, y=w2043) -> (x-y=w2041:i32)
                    n726 = call "FindRobotByID.vi"("id"=w2041, "RobotRef"=w2045) -> ("index"=w2048:i32, "Robot"=w2044:refnum<class "Robot.lvclass">)  [unwired: 6 in, 2 out]
                    n727 = Not Equal?(x=w2048, y=-1) -> (x != y?=w2046:bool)
                  }
                  n728 = for {
                    tunnel: w2022 -> [w2033] mode=indexing
                    tunnel: w2023 -> [w2032]
                    tunnel: w2022 -> [w2029]
                    tunnel: [w2026] -> w2021
                    i -> [w2028]
                    stop <- w2025 stop-if-true
                    n729 = property class="Robot"(reference=w2033) -> ("id"=w2031:i32)  [unwired: 1 in, 2 out]
                    n730 = property class="Robot"(reference=w2032) -> (reference out=w2027:refnum<class "Robot.lvclass">, "id"=w2030:i32)  [unwired: 1 in, 1 out]
                    n731 = Equal?(x=w2031, y=w2030) -> (x = y?=w2025:bool)
                    n732 = case shown="True" w2025 {
                      tunnel: w2029 -> [w2034 w2040]
                      tunnel: [w2034 w2039] -> w2026
                      tunnel: w2028 -> [_ w2038]
                      tunnel: w2027 -> [_ w2037]
                      frame False {
                      }
                      frame True {
                        n733 = property class="Robot"(reference=w2037, "role"=roles."AttackerAimGoal") -> (reference out=w2035:refnum<class "Robot.lvclass">)  [unwired: 1 in, 1 out]
                        n734 = Replace Array Subset(array=w2040, new element=w2035, index=w2038) -> (w2039:refnum<class "Robot.lvclass">[])
                      }
                    }
                  }
                }
                frame True {
                }
              }
            }
            frame "KickPenaltyAlly" {
              n735 = Unbundle By Name(w2079) -> ("AllyTeamArray"=w2078:T4[], "ShootOutRobotId"=w2073:dbl)
              n736 = call "PickActiveTeam.vi"("Robots"=w2080, "AllyTeamArray"=w2078, "Team"=AllyTeam."Attacker") -> ("Robots out"=w2075:refnum<class "Robot.lvclass">[])  [unwired: 15 in, 1 out]
              n737 = call "PickActiveTeam.vi"("Robots"=w2080, "AllyTeamArray"=w2078, "Team"=AllyTeam."Defender") -> ("Robots out"=w2081:refnum<class "Robot.lvclass">[])  [unwired: 15 in, 1 out]
              n738 = Insert Into Array(array=w2075, new element=w2081) -> (w2074:refnum<class "Robot.lvclass">[])  [unwired: 1 in]
              n739 = for {
                tunnel: w2074 -> [w2123] mode=indexing
                tunnel: w2073 -> [w2121]
                tunnel: [w2118] -> w2069 mode=indexing
                shift-right: [w2113] -> w2068
                shift-left: FALSE -> [w2114]
                n740 = property class="Robot"(reference=w2123) -> (reference out=w2119:refnum<class "Robot.lvclass">, "id"=w2122:i32)  [unwired: 1 in, 1 out]
                n741 = To Long Integer(number=w2121) -> (32bit integer=w2120:i32)
                n742 = Equal?(x=w2122, y=w2120) -> (x = y?=w2112:bool)
                n743 = Select(t=roles."PenaltyAttacker" ("role"), s=w2112, f=roles."Halt" ("role")) -> (s? t:f=w2115:T5)
                n744 = property class="Robot"(reference=w2119, "role"=w2115) -> (reference out=w2118:refnum<class "Robot.lvclass">)  [unwired: 1 in, 1 out]
                n745 = Select(t=TRUE, s=w2112, f=w2114) -> (s? t:f=w2113:bool)
              }
              n746 = case shown="False" w2068 {
                tunnel: w2069 -> [w2083 w2110]
                tunnel: [w2082 w2110] -> w2067
                frame False {
                  n747 = for {
                    N: 6 -> [_]
                    tunnel: w2083 -> [w2106]
                    tunnel: [w2105] -> w2084
                    i -> [w2104]
                    stop <- w2107 stop-if-true
                    n748 = Subtract(x=5, y=w2104) -> (x-y=w2102:i32)
                    n749 = call "FindRobotByID.vi"("id"=w2102, "RobotRef"=w2106) -> ("index"=w2109:i32, "Robot"=w2105:refnum<class "Robot.lvclass">)  [unwired: 6 in, 2 out]
                    n750 = Not Equal?(x=w2109, y=-1) -> (x != y?=w2107:bool)
                  }
                  n751 = for {
                    tunnel: w2083 -> [w2094] mode=indexing
                    tunnel: w2084 -> [w2093]
                    tunnel: w2083 -> [w2090]
                    tunnel: [w2087] -> w2082
                    i -> [w2089]
                    stop <- w2086 stop-if-true
                    n752 = property class="Robot"(reference=w2094) -> ("id"=w2092:i32)  [unwired: 1 in, 2 out]
                    n753 = property class="Robot"(reference=w2093) -> (reference out=w2088:refnum<class "Robot.lvclass">, "id"=w2091:i32)  [unwired: 1 in, 1 out]
                    n754 = Equal?(x=w2092, y=w2091) -> (x = y?=w2086:bool)
                    n755 = case shown="True" w2086 {
                      tunnel: w2090 -> [w2095 w2101]
                      tunnel: [w2095 w2100] -> w2087
                      tunnel: w2089 -> [_ w2099]
                      tunnel: w2088 -> [_ w2098]
                      frame False {
                      }
                      frame True {
                        n756 = property class="Robot"(reference=w2098, "role"=roles."PenaltyAttacker") -> (reference out=w2096:refnum<class "Robot.lvclass">)  [unwired: 1 in, 1 out]
                        n757 = Replace Array Subset(array=w2101, new element=w2096, index=w2099) -> (w2100:refnum<class "Robot.lvclass">[])
                      }
                    }
                  }
                }
                frame True {
                }
              }
            }
            frame "SimplePass" {
              w2174 = 1.0 ("y")
              # "id receiver"
              # "id passer"
              # "TIRAR DPS"
              # "Para fixar o receiver"
              # "firstCall"
              n758 = Absolute Value(x=w2162) -> (abs(x)=w2161:dbl)
              n759 = Absolute Value(x=w2160) -> (abs(x)=w2159:dbl)
              n760 = Unbundle By Name(w2140) -> ("AllyTeamArray"=w2139:T4[])
              n761 = Greater?(x=w2159, y=w2174) -> (0:w2172:bool)
              n762 = Greater?(x=w2161, y=w2174) -> (0:w2173:bool)
              n763 = Or(x=w2173, y=w2172) -> (x .or. y?=w2170:bool)
              n764 = call "PickActiveTeam.vi"("Robots"=w2141, "AllyTeamArray"=w2139, "Team"=AllyTeam."Attacker") -> ("Robots out"=w2130:refnum<class "Robot.lvclass">[])  [unwired: 15 in, 1 out]
              n765 = property class="Ally"(reference=w2129) -> ("RobotRef"=w2133:refnum<class "Robot.lvclass">[])  [unwired: 1 in, 2 out]
              n766 = Array Size(array=w2130) -> (size(s)=w2132:i32)
              n767 = call "UpdateZones.vi"("Old Robots"=w2133, "object in"=w2127) -> ("object out"=w2125:refnum<class "Ally.lvclass">)  [unwired: 8 in, 1 out]
              n768 = call "ChooseZones.vi"("NumberOfAttackers"=w2132, "Game"=w2131, "object in"=w2125) -> ("Zones"=w2128:refnum<class "Zone.lvclass">[], "object out"=w2126:refnum<class "Ally.lvclass">)  [unwired: 6 in, 1 out]
              n769 = property class="Ball"(reference=w2144) -> ("x"=w2147:dbl, "y"=w2146:dbl, "position(x,y)"=w2145:dbl[])  [unwired: 1 in, 2 out]
              n770 = Not(x=w2170) -> (.not. x?=w2171:bool)
              n771 = feedback #14() -> (w2169:i32)  [unwired: 1 in]
              n772 = case shown="True" w2171 {
                tunnel: w2158 -> [_ w2232]
                tunnel: w2130 -> [_ w2231]
                tunnel: [w2225 w2228] -> w2134
                tunnel: w2169 -> [w2225 _]
                tunnel: w2147 -> [_ w2227]
                tunnel: w2146 -> [_ w2226]
                frame False {
                }
                frame True {
                  n773 = for {
                    tunnel: w2231 -> [w2248] mode=indexing
                    shift-right: [w2241] -> w2228
                    shift-left: -2 ("id") -> [w2237]
                    shift-right: [w2239] -> _
                    shift-left: inf -> [w2236]
                    tunnel: w2232 -> [w2235]
                    tunnel: w2227 -> [w2234]
                    tunnel: w2226 -> [w2233]
                    n774 = property class="Robot"(reference=w2248) -> ("id"=w2240:i32, "x"=w2247:dbl, "y"=w2246:dbl)  [unwired: 1 in, 2 out]
                    n775 = Build Array(w2234, w2233) -> (w2244:dbl[])
                    n776 = Build Array(w2247, w2246) -> (w2245:dbl[])
                    n777 = Subtract(x=w2245, y=w2244) -> (x-y=w2243:dbl[])
                    n778 = call "Module.vi"("2D vector"=w2243, "Utilities in"=w2235) -> ("Modulo"=w2238:dbl)  [unwired: 7 in, 2 out]
                    n779 = Less?(x=w2238, y=w2236) -> (x < y?=w2242:bool)
                    n780 = case shown="True" w2242 {
                      tunnel: [w2250 w2252] -> w2241
                      tunnel: w2240 -> [_ w2252]
                      tunnel: [w2249 w2251] -> w2239
                      tunnel: w2238 -> [_ w2251]
                      tunnel: w2237 -> [w2250 _]
                      tunnel: w2236 -> [w2249 _]
                      frame False {
                      }
                      frame True {
                      }
                    }
                  }
                }
              }
              n781 = feedback-in #14(w2134) -> ()
              n782 = property class="Game"(reference=w2131) -> ("Playbook"=w2190:refnum<class "Playbook.lvclass">)  [unwired: 1 in, 2 out]
              n783 = property class="Playbook"(reference=w2190) -> ("offensive_plays"=w2189:T10)  [unwired: 1 in, 2 out]
              n784 = Unbundle By Name(w2189) -> ("5RobotsPassGamePlay"=w2188:refnum<class "5RobotsPassGamePlay.lvclass">)
              n785 = property class="5RobotsPassGamePlay"(reference=w2188) -> ("FactorPass"=w2187:cluster{"id":dbl[], "value":dbl[]})  [unwired: 1 in, 2 out]
              n786 = property class="Game"(reference=w2131) -> ("Parameters.lvclass"=w2157:refnum<class "Parameters.lvclass">, "Referee"=w2155:refnum<class "Referee.lvclass">)  [unwired: 1 in, 2 out]
              n787 = property class="Referee"(reference=w2155) -> ("our_goalie_id"=w2154:i32)  [unwired: 1 in, 2 out]
              n788 = property class="Parameters.lvclass"(reference=w2157) -> ("minDistanceToPass"=w2156:dbl)  [unwired: 1 in, 2 out]
              n789 = Unbundle By Name(w2187) -> ("id"=w2138:dbl[], "value"=w2184:dbl[])
              n790 = To Long Integer(number=w2138) -> (32bit integer=w2137:i32[])
              n791 = for {
                tunnel: w2184 -> [w2274] mode=indexing
                shift-right: [w2271] -> w2179
                shift-left: -1 ("id") -> [w2273]
                shift-right: [w2270] -> _
                shift-left: -1.0 -> [w2272]
                tunnel: [w2270] -> _ mode=indexing
                tunnel: w2137 -> [w2259] mode=indexing
                tunnel: w2144 -> [w2264]
                tunnel: w2158 -> [w2263]
                tunnel: w2156 -> [w2262]
                tunnel: w2154 -> [w2261]
                tunnel: w2130 -> [w2260]
                tunnel: w2134 -> [w2257]
                n792 = call "FindRobotByID.vi"("id"=w2259, "RobotRef"=w2260) -> ("Robot"=w2258:refnum<class "Robot.lvclass">)  [unwired: 6 in, 3 out]
                n793 = call "distanceRobotToBall.vi"("Robot"=w2258, "Ball"=w2264, "Utilities in"=w2263) -> ("Distance Robot To Ball"=w2266:dbl)  [unwired: 6 in, 2 out]
                n794 = Equal?(x=w2259, y=w2261) -> (x = y?=w2267:bool)
                n795 = Equal?(x=w2257, y=w2259) -> (x = y?=w2269:bool)
                n796 = Less Or Equal?(x=w2266, y=w2262) -> (x <= y?=w2265:bool)
                n797 = Compound Arithmetic op=OR(w2267, w2269, w2265) -> (w2268:bool)
                n798 = case shown="False" w2268 {
                  tunnel: [w2275 w2283] -> w2271
                  tunnel: w2274 -> [w2281 _]
                  tunnel: w2273 -> [w2277 w2283]
                  tunnel: w2272 -> [w2279 w2282]
                  tunnel: [w2280 w2282] -> w2270
                  tunnel: w2259 -> [w2276 _]
                  frame False {
                    n799 = Greater?(x=w2281, y=w2279) -> (0:w2278:bool)
                    n800 = Select(t=w2281, s=w2278, f=w2279) -> (s? t:f=w2280:dbl)
                    n801 = Select(t=w2276, s=w2278, f=w2277) -> (s? t:f=w2275:i32)
                  }
                  frame True {
                  }
                }
              }
              n802 = Not(x=w2150) -> (.not. x?=w2151:bool)
              n803 = feedback #15(-2 ("id")) -> (w2167:i32)
              n804 = Equal?(x=0, y=w2167) -> (x = y?=w2177:bool)
              n805 = Equal?(x=-1, y=w2167) -> (x = y?=w2166:bool)
              n806 = Not(x=w2166) -> (.not. x?=w2165:bool)
              n807 = Not(x=w2177) -> (.not. x?=w2163:bool)
              n808 = And(x=w2165, y=w2163) -> (x .and. y?=w2164:bool)
              n809 = feedback #16(-1 ("id")) -> (w2180:i32)
              n810 = Equal?(x=w2134, y=w2180) -> (x = y?=w2175:bool)
              n811 = And(x=w2175, y=w2164) -> (x .and. y?=w2153:bool)
              n812 = And(x=w2151, y=w2153) -> (x .and. y?=w2152:bool)
              n813 = case shown="False" w2152 {
                tunnel: w2179 -> [w2253 _]
                tunnel: [w2253 w2256] -> w2136
                tunnel: w2134 -> [w2254 _]
                tunnel: [w2254 w2255] -> w2183
                tunnel: [w2253 w2256] -> w2181
                tunnel: w2167 -> [_ w2256]
                tunnel: w2180 -> [_ w2255]
                frame False {
                }
                frame True {
                }
              }
              n814 = for {
                tunnel: w2130 -> [w2217] mode=indexing
                tunnel: w2136 -> [w2216]
                tunnel: [w2213] -> w2135 mode=indexing
                tunnel: w2134 -> [w2205]
                tunnel: w2128 -> [w2204] mode=indexing
                n815 = property class="Robot"(reference=w2217) -> (reference out=w2214:refnum<class "Robot.lvclass">, "id"=w2210:i32)  [unwired: 1 in, 1 out]
                n816 = Equal?(x=w2210, y=w2216) -> (x = y?=w2215:bool)
                n817 = Equal?(x=w2210, y=w2205) -> (x = y?=w2209:bool)
                n818 = Select(t=roles."PassBestRobot" ("role"), s=w2209, f=roles."5Robots1st" ("role")) -> (s? t:f=w2207:T5)
                n819 = Select(t=roles."PassBestReceiver" ("role"), s=w2215, f=w2207) -> (s? t:f=w2211:T5)
                n820 = property class="Robot"(reference=w2214, "role"=w2211, "Zone"=w2204) -> (reference out=w2213:refnum<class "Robot.lvclass">)  [unwired: 1 in, 1 out]
              }
              n821 = feedback-in #15(w2181) -> ()
              n822 = feedback-in #16(w2183) -> ()
              n823 = call-dynamic "5RobotsPosition.vi"("Game"=w2131, "Utilities in"=w2158) -> ("5Positions"=w2149:dbl[][])  [unwired: 7 in, 2 out]
              n824 = disable-structure shown="Enabled" {
                disable-tunnel: w2149 -> [w2223 w2224]
                disable-tunnel: w2135 -> [w2221 _]
                disable-tunnel: [w2219 w2224] -> w2148
                disable-tunnel: w2145 -> [w2218 _]
                frame Disabled {
                  n825 = call "eliminatePositionRobot.vi"("position(x,y)"=w2218, "5Positions"=w2223) -> ("sorted 2D array"=w2222:dbl[][])  [unwired: 9 in]
                  n826 = property class="Robot"(reference=w2221) -> ("position(x,y)"=w2220:dbl[])  [unwired: 1 in, 2 out]
                  n827 = call "eliminatePositionRobot.vi"("position(x,y)"=w2220, "5Positions"=w2222) -> ("sorted 2D array"=w2219:dbl[][])  [unwired: 9 in]
                }
                frame Enabled {
                }
              }
              n828 = disable-structure shown="Enabled" {
                disable-tunnel: w2148 -> [w2194 _]
                disable-tunnel: [w2193 w2203] -> w2143
                disable-tunnel: w2135 -> [w2192 w2203]
                disable-tunnel: w2131 -> [w2191 _]
                frame Disabled {
                  n829 = for {
                    tunnel: refnum<class "5RobotsSkill.lvclass"> refnum ("5RobotsSkill in") -> [w2202]
                    tunnel: [w2197] -> w2193 mode=indexing
                    tunnel: w2191 -> [w2201]
                    tunnel: w2194 -> [w2200]
                    tunnel: w2192 -> [w2196] mode=indexing
                    i -> [w2199]
                    n830 = call-dynamic "5RobotsSkill.vi"("Eliminate"=EliminateEnum."2", "id"=w2199, "5Positions"=w2200, "Robot In"=w2196, "Game in"=w2201, "5RobotsSkill in"=w2202) -> ("Robot out"=w2197:refnum<class "Robot.lvclass">)  [unwired: 3 in, 2 out]
                  }
                }
                frame Enabled {
                }
              }
            }
            frame "5RobotsKeeperGame" {
              w2322 = 1.0 ("y")
              # "new offensive team"
              n831 = Absolute Value(x=w2315) -> (abs(x)=w2314:dbl)
              n832 = Absolute Value(x=w2313) -> (abs(x)=w2312:dbl)
              n833 = case shown="5, 6, Default" w2337 {
                tunnel: [0 ("number_of_robots") 1 w2354 w2360] -> w2341
                tunnel: w2336 -> [_ _ w2355 w2359]
                tunnel: w2338 -> [_ _ w2351 w2358]
                frame 0, 1 {
                }
                frame 2, 3 {
                }
                frame 4 {
                  n834 = Subtract(x=w2351, y=2) -> (x-y=w2352:i32)
                  n835 = Equal?(x=w2355, y=2) -> (x = y?=w2356:bool)
                  n836 = Select(t=w2355, s=w2356, f=w2352) -> (s? t:f=w2354:i32)
                }
                frame 5, 6, Default {
                  n837 = Less?(x=w2358, y=w2359) -> (x < y?=w2361:bool)
                  n838 = Select(t=w2358, s=w2361, f=w2359) -> (s? t:f=w2360:i32)
                }
              }
              n839 = Greater?(x=w2312, y=w2322) -> (0:w2320:bool)
              n840 = Greater?(x=w2314, y=w2322) -> (0:w2321:bool)
              n841 = Or(x=w2321, y=w2320) -> (x .or. y?=w2302:bool)
              n842 = Array Subset(array=w2340, index=w2339, length=w2341) -> (w2310:refnum<class "Robot.lvclass">[])
              n843 = property class="Game"(reference=w2293) -> ("Playbook"=w2335:refnum<class "Playbook.lvclass">)  [unwired: 1 in, 2 out]
              n844 = property class="Playbook"(reference=w2335) -> ("offensive_plays"=w2334:T10)  [unwired: 1 in, 2 out]
              n845 = Unbundle By Name(w2334) -> ("5RobotsKeeperGame"=w2333:refnum<class "5RobotsKeeperGame.lvclass">)
              n846 = property class="5RobotsKeeperGame"(reference=w2333) -> ("FactorPass"=w2332:cluster{"id":dbl[], "value":dbl[]})  [unwired: 1 in, 2 out]
              n847 = Unbundle By Name(w2332) -> ("id"=w2329:dbl[], "value"=w2328:dbl[])
              n848 = for {
                tunnel: w2328 -> [w2375] mode=indexing
                shift-right: [w2372] -> w2305
                shift-left: -1 ("id") -> [w2374]
                shift-right: [w2371] -> _
                shift-left: -1.0 -> [w2373]
                tunnel: [w2371] -> _ mode=indexing
                tunnel: w2329 -> [w2370] mode=indexing
                n849 = Equal?(x=w2370, y=0.0) -> (x = y?=w2368:bool)
                n850 = case shown="True" w2368 {
                  tunnel: [w2376 w2384] -> w2372
                  tunnel: w2375 -> [w2382 _]
                  tunnel: w2374 -> [w2378 w2384]
                  tunnel: w2373 -> [w2380 w2383]
                  tunnel: [w2381 w2383] -> w2371
                  tunnel: w2370 -> [w2377 _]
                  frame False {
                    n851 = Greater?(x=w2382, y=w2380) -> (0:w2379:bool)
                    n852 = Select(t=w2382, s=w2379, f=w2380) -> (s? t:f=w2381:dbl)
                    n853 = Select(t=w2377, s=w2379, f=w2378) -> (s? t:f=w2376:dbl)
                  }
                  frame True {
                  }
                }
              }
              n854 = feedback #17(-2.0 ("id")) -> (w2304:dbl)
              n855 = Not Equal?(x=w2305, y=w2304) -> (x != y?=w2303:bool)
              n856 = Equal?(x=0.0, y=w2304) -> (x = y?=w2324:bool)
              n857 = Equal?(x=w2304, y=-2.0) -> (x = y?=w2308:bool)
              n858 = Equal?(x=-1.0, y=w2304) -> (x = y?=w2318:bool)
              n859 = Not(x=w2318) -> (.not. x?=w2317:bool)
              n860 = Not(x=w2324) -> (.not. x?=w2316:bool)
              n861 = And(x=w2303, y=w2302) -> (x .and. y?=w2301:bool)
              n862 = Not(x=w2308) -> (.not. x?=w2307:bool)
              n863 = And(x=w2317, y=w2316) -> (x .and. y?=w2306:bool)
              n864 = Not(x=w2301) -> (.not. x?=w2299:bool)
              n865 = And(x=w2307, y=w2306) -> (x .and. y?=w2298:bool)
              n866 = And(x=w2299, y=w2298) -> (x .and. y?=w2300:bool)
              n867 = case shown="True" w2300 {
                tunnel: w2305 -> [w2366 _]
                tunnel: [w2366 w2367] -> w2327
                tunnel: [w2366 w2367] -> w2326
                tunnel: w2304 -> [_ w2367]
                frame False {
                }
                frame True {
                }
              }
              n868 = feedback-in #17(w2326) -> ()
              n869 = call "DeleteRobotByID.vi"("id"=w2327, "RobotRef"=w2310, "Utilities in"=w2297) -> ("RobotRef out"=w2287:refnum<class "Robot.lvclass">[])  [unwired: 6 in, 2 out]
              n870 = call "FindRobotByID.vi"("id"=w2327, "RobotRef"=w2310, "Utilities in"=w2297) -> ("index"=w2296:i32, "Robot"=w2291:refnum<class "Robot.lvclass">)  [unwired: 5 in, 2 out]
              n871 = Equal?(x=w2296, y=-1) -> (x = y?=w2294:bool)
              n872 = case shown="False" w2294 {
                tunnel: w2291 -> [_ w2365]
                tunnel: refnum<class "Robot.lvclass">[] [] -> [w2362 w2364]
                tunnel: [w2362 w2363] -> w2288
                frame True {
                }
                frame False {
                  n873 = Insert Into Array(array=w2364, new element=w2365) -> (w2363:refnum<class "Robot.lvclass">[])  [unwired: 1 in]
                }
              }
              n874 = call-dynamic "5RobotsPosition.vi"("Game"=w2293, "Utilities in"=w2297) -> ("5Positions"=w2290:dbl[][])  [unwired: 7 in, 2 out]
              n875 = Insert Into Array(array=w2288, new element=w2287) -> (w2286:refnum<class "Robot.lvclass">[])  [unwired: 1 in]
              n876 = for {
                tunnel: w2286 -> [w2344] mode=indexing
                tunnel: w2290 -> [w2348]
                tunnel: w2293 -> [w2347]
                tunnel: refnum<class "5RobotsSkill.lvclass"> refnum ("5RobotsSkill in") -> [w2346]
                tunnel: [w2345] -> w2289 mode=indexing
                i -> [w2343]
                n877 = call-dynamic "5RobotsSkill.vi"("Eliminate"=EliminateEnum."0", "id"=w2343, "5Positions"=w2348, "Robot In"=w2344, "Game in"=w2347, "5RobotsSkill in"=w2346) -> ("Robot out"=w2345:refnum<class "Robot.lvclass">)  [unwired: 3 in, 2 out]
              }
            }
          }
          n878 = feedback-in #3(w83) -> ()
        }
      }
      n879 = call "updateDest.vi"("NewAllyRobots"=w36, "LastAlly"=w35) -> ("NewAllyRobotsUpdated"=w37:refnum<class "Robot.lvclass">[])  [unwired: 7 in, 2 out]
      n880 = property class="Ally"(reference=w20, "RobotRef"=w37) -> (reference out=w47:refnum<class "Ally.lvclass">)  [unwired: 1 in, 1 out]
    }
    frame Error {
    }
  }
  "error out" <- w11
  "OffensiveTeam out" <- w13
  "RobotRef" <- w6
